vi "plcHMI.vi"() -> ()   [LabVIEW 2020]
doc: "ADS continuos synchronous write example using base blocks. \n\nThe client writes data synchronously and does wait for the respose from server."
uses:
  Agilent/AgilentTotalCluster.ctl
  Agilent/AgilentControl.ctl
  Agilent/Channel Config.ctl
  <vilib>/Platform/TimedLoop/XDataNode/timing_clust.ctl
  <vilib>/Platform/TimedLoop/XDataNode/nitl_modes.ctl
  <vilib>/Platform/TimedLoop/XDataNode/wakeup.ctl
  <userlib>/Beckhoff-LabVIEW-Interface/_DependsOn/With TypeResolving/Write Sync Single TypeResolved.vi
  <userlib>/Beckhoff-LabVIEW-Interface/_DependsOn/With TypeResolving/Read Sync Single TypeResolved.vi
  <vilib>/platform/TimedLoop/XDataNode/XDataNode.xnode
  <vilib>/Platform/TimedLoop/XDataNode/XDNodeRunTimeDep.lvlib
panel:
  in  "Tab Control":T1(tab)
  out "error out":errorcluster
  in  "Symbol file path - MUST BE ENTERED\nLoad \"ADS Write AND Read Symbols REV X.X.xml\"":path
  out "bHasMached":bool
  out "Write Status":bool
  out "Read Status":bool
  in  "EXIT HMI":bool caption="STOP HMI\nEXIT HMI"
  out "Internal TwinCAT Handle ID Maps":dbl format="%#_12g"
  in  "802L TDK PSU Voltage Rating (abs(Volts))":i32=12000 min=1 max=50000
  in  "802L TDL PSU Peak Power (J/s)":i32=9000 min=1 max=50000
  in  "HVPS Model":u16(ring) items=["802L-12kV,9000J/s", "802L+50kV,9000J/s", "Other"]
  in  "Voltage Held by PSU":bool
  in  "Log Capacitor Voltage":bool
  in  "Log Temperature Data":bool
  out "Time Since Last Shot":string caption="Elapsed Time Text"
  in  "Duty Cycle":dbl
  in  "Current Control":bool
  out "Expected Voltage":i16
  in  "Dump":bool
  out "EOC":bool
  out "Maximum Test Number Reached":bool
  out "SCR Ready":bool
  in  "START":bool
  in  "STOP":bool
  in  "Hold":bool
  in  "Charge":bool
  in  "Shot":bool
  in  "HV Switch Mode":bool
  in  "CLEAR FAULT":bool
  in  "Manual/Auto":bool=TRUE
  in  "Cycle Time (seconds)":i32=15 min=0
  in  "Capacitance (uF)":sgl=1e-13 min=0 max=10000 format="%#_6f"
  in  "Target Charge Volt (V) - Min 1500V - TEMPORARY LIMIT 12kV":i32 min=-12000 max=12000 step=1
  out "Estimated Charge Time (seconds)":sgl
  in  "Hold Time Before Shot (seconds)":i16 min=0 max=1000
  in  "Max Number of Shots (Test intervals)":i32=1 min=1 max=999
  out "Shot Number":i32
  out "Charge Fault":bool=TRUE
  out "Discharge Fault":bool=TRUE
  out "Hold Fault":bool=TRUE
  out "Cap 1 Temp\nExceeded Fault":bool=TRUE
  out "Ambient Temp\nExceeded Fault":bool=TRUE
  out "PSU Fault":bool=TRUE
  out "Control Sys Fault":bool=TRUE
  out "test Running":bool
  out "Test State":string
  out "Cap 1 Voltage":i16
  out "Cap 1 Temperature":i16
  in  "Capacitor Voltage Data Log File Path (.xlsx)":path
  out "Load Temperature":i16
  out "Soft Dump Temp":i16
  out "Ambient Temp":i16
  out "Waveform Chart - Capacitor Voltage (Probe, abs(Volts))":dbl(graph)
  in  "Manual Charge Time (seconds)":sgl=-1.0 min=-1 max=90
  in  "Reset Test Number":bool
  in  "Cap 1 Fault Temp (Cel)":i16 min=0 max=125
  in  "Capacitor Temperature Data Log File Path (.xlsx)":path
  out "Cap 1 Voltage (HVPS)":i16
  out "Capacitor Voltage":cluster{dbl, dbl}(graph)
  out "EOC":i16(graph)
  out "Soft Exception":bool
  out "PSU HV FB Fault":bool
  out "Charge FB Fault":bool
  out "Softdump FB Fault":bool
  out "SCR FB":i16(graph)
  in  "CH4 Vertical Units":string(combo)="V"
  in  "CH4 Vertical Units/div":dbl=2.0
  in  "Toggle Scope Scale":bool
  in  "CH1 Vertical Units/div":dbl=2.0
  in  "CH1 Vertical Units":string(combo)="V"
  in  "Horizontal Units":enum16{"us", "ms", "s"}(ring)
  in  "Horizontal Units/div":dbl=200.0
  out "Download":bool
  in  "Single":bool
  in  "Stop":bool
  out "Scope Trig":bool
  in  "Agilent Array":T2[](array[typedef])
  out "Process Step":i32
  out "Stop Loops":bool
  # "CONFIGURATION"
  # "Press STOP HMI instead of\nLabView Abort Execution"
  # "PSU V Rating, Peak Power\nactive when OTHER\nis selected"
  # "INPUT VARIABLES - For TDK Lambda 802L\nMust be written to before START"
  # "FAULT STATUSES"
  # "Set to -1 for automated\nfull charge to setpoint"
  # "MANUAL CONTROLS"
  # "Does not record during \"wait\" and appends to data file. Must be named with .xlsx"
  # "HV Switch Configuration"
  # "Records during \"Test Running.\" Must be named with .xlsx"
  # "Control Sys Faults"
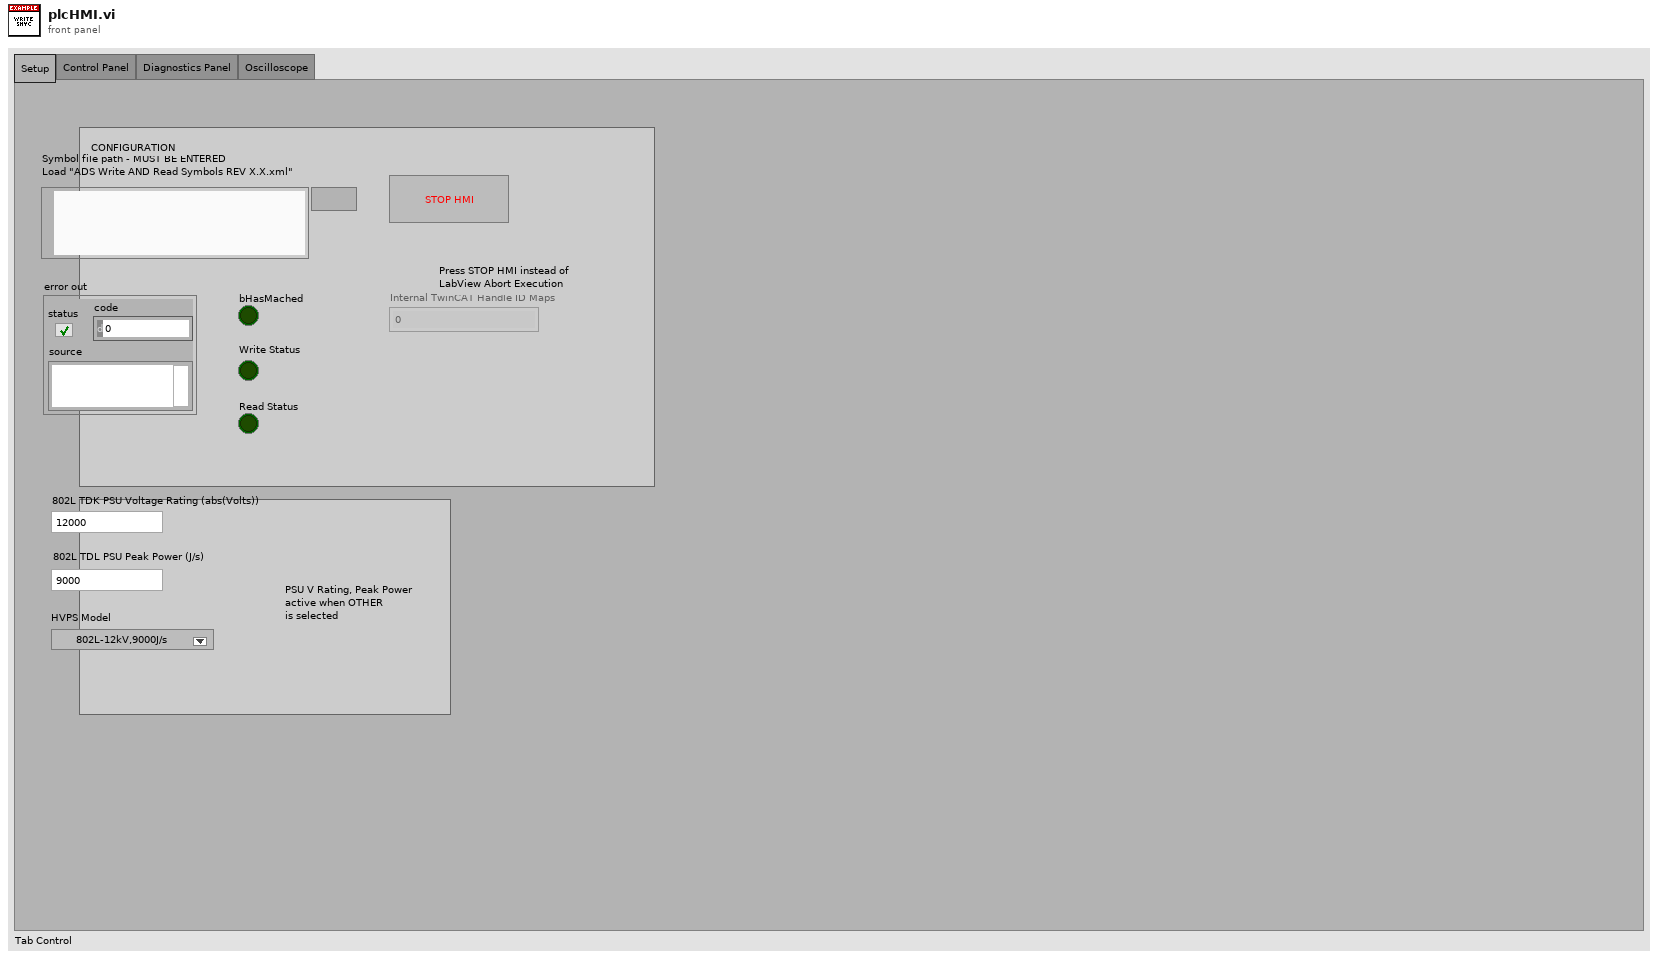
[diagram p1: front panel]
types:
  T1 = enum32{"Setup", "Control Panel", "Diagnostics Panel", "Oscilloscope"}
  T2 = typedef "AgilentTotalCluster.ctl" = cluster{"Agilent Graph":waveform(dbl)[], "Agilent Control":T3, "Agilent Setup Error":errorcluster, "Agilent Present":bool, "Enabled":bool}
  T3 = typedef "AgilentControl.ctl" = cluster{"Trig?":bool, "VISA session":refnum<visa-resource-name>, "Setup to Load":string, "Timeout (ms)":u32, "Desired Samp":enum32{"100", "250", "500", "1000", "2000", "5000", "10000", "20000", "50000", "100000", "200000", "500000", "1000000", "2000000", "4000000", "8000000"}, "Captured Samp":i32, "Desired Channels":T4[]}
  T4 = typedef "Channel Config.ctl" = cluster{"Chan Index":enum16{"Channel1", "Channel2", "Channel3", "Channel4", "MATH"}, "Name":string, "Samples":i32}
  T5 = typedef "XDNodeRunTimeDep.lvlib/timing_clust.ctl" = cluster{"Expected End [f-1]":u64, "Actual End [f-1]":u64, "Finished Late? [f-1]":bool, "Expected End [i-1]":u64, "Actual End [i-1]":u64, "Finished Late? [i-1]":bool, "Expected Start [i]":u64, "Actual Start [i]":u64, "Expected Start [f]":u64, "Actual Start [f]":u64, "Source Name":string, "Structure Name":string, "Period":i64, "Deadline":i64, "Offset":i64, "Start":i64, "Priority":i32, "Timeout":i32, "Mode":T6, "Wakeup Reason":T7, "Error":errorcluster, "Source Type":string, "Secondary Source Type":string, "Global End Time":u64, "Global Start Time":u64, "Frame Duration":u64, "Iteration Duration":u64, "Assigned CPU":i32, "I/O Scan Engine Mode":u32}
  T6 = typedef "XDNodeRunTimeDep.lvlib/nitl_modes.ctl" = enum32{"No Change", "Process missed periods, maintain original phase", "Discard missed periods, maintain original phase", "Process missed periods, ignore original phase", "Discard missed periods, ignore original phase"}
  T7 = typedef "XDNodeRunTimeDep.lvlib/wakeup.ctl" = enum32{"Normal", "Aborted", "Asynchronous wakeup", "Timing source error", "Timed loop error", "Timeout"}
  T8 = cluster{"Agilent Array[0]":T2, "Agilent Array[1]":T2, "Agilent Array[2]":T2, "Agilent Array[3]":T2, "Agilent Array[4]":T2, "Agilent Array[5]":T2, "Agilent Array[6]":T2, "Agilent Array[7]":T2, "Agilent Array[8]":T2}
  T9 = enum32{"100", "250", "500", "1000", "2000", "5000", "10000", "20000", "50000", "100000", "200000", "500000", "1000000", "2000000", "4000000", "8000000"}
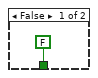
[diagram p2: hidden frame]
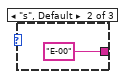
[diagram p5: hidden frame]
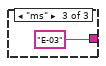
[diagram p6: hidden frame]
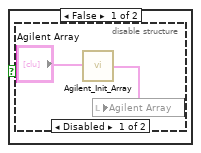
[diagram p7: hidden frame]
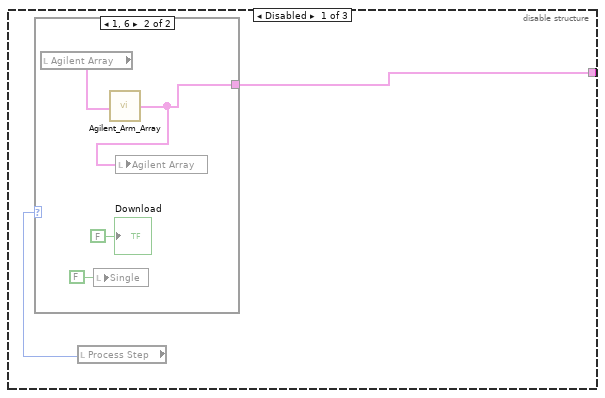
[diagram p11: hidden frame]
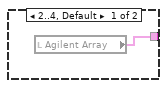
[diagram p12: hidden frame]
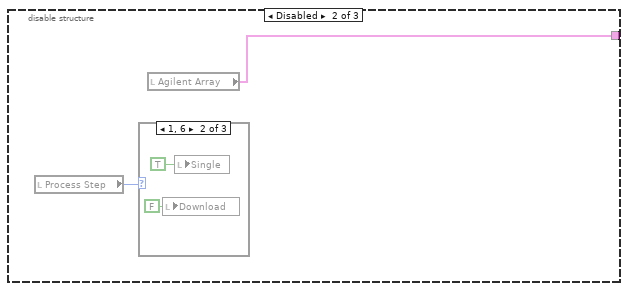
[diagram p13: hidden frame]
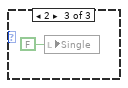
[diagram p15: hidden frame]
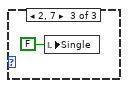
[diagram p17: hidden frame]
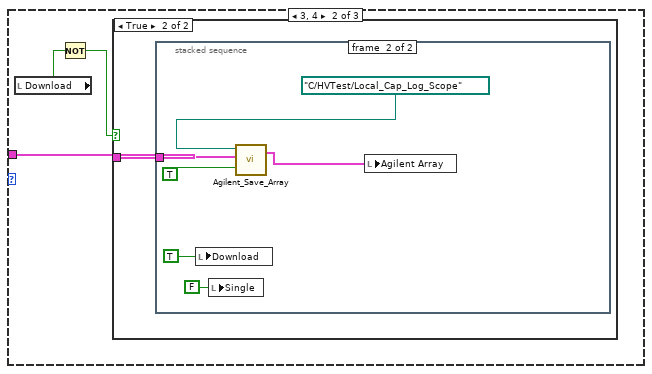
[diagram p19: hidden frame]
diagram:
  w89 = u16 17 items=["SyncLatest"=17, "AsyncLatest"=33] ("WriterMode")
  w182 = u16 33 items=["SyncLatest"=17, "AsyncLatest"=33] ("WriterMode")
  w221 = u16 33 items=["SyncLatest"=17, "AsyncLatest"=33] ("WriterMode")
  w240 = u16 33 items=["SyncLatest"=17, "AsyncLatest"=33] ("WriterMode")
  w259 = u16 33 items=["SyncLatest"=17, "AsyncLatest"=33] ("WriterMode")
  w278 = u16 33 items=["SyncLatest"=17, "AsyncLatest"=33] ("WriterMode")
  w297 = u16 33 items=["SyncLatest"=17, "AsyncLatest"=33] ("WriterMode")
  w316 = u16 33 items=["SyncLatest"=17, "AsyncLatest"=33] ("WriterMode")
  w335 = u16 17 items=["SyncLatest"=17, "AsyncLatest"=33] ("WriterMode")
  w354 = u16 17 items=["SyncLatest"=17, "AsyncLatest"=33] ("WriterMode")
  w373 = u16 17 items=["SyncLatest"=17, "AsyncLatest"=33] ("WriterMode")
  w392 = u16 17 items=["SyncLatest"=17, "AsyncLatest"=33] ("WriterMode")
  w411 = u16 17 items=["SyncLatest"=17, "AsyncLatest"=33] ("WriterMode")
  w430 = u16 17 items=["SyncLatest"=17, "AsyncLatest"=33] ("WriterMode")
  w449 = u16 17 items=["SyncLatest"=17, "AsyncLatest"=33] ("WriterMode")
  w464 = u16 17 items=["SyncLatest"=17, "AsyncLatest"=33] ("WriterMode")
  # "Variables/ Control"
  # "Documentation:\nCode separated vertically into two main sections - Write and read\nThey are further separated into BOOL and numeric\nThe OR gates wire all the error lines and the EXIT HMI button to a WHILE LOOP STOP\nThere current delay time on the routine is 100ms\nAll the AND gates connect the typecast resolve lines to the bHasMatched indicator\nThe second and third set of AND gates connect the write statuses to the Write Status indicator\nThe same is done for the read status indicator"
  # "WRITE NUMERICS"
  # "WRITE BOOLS"
  # "Select Symbol N"
  # "Read Initialization"
  # "Release \nTypeResolver"
  # "Release Writer"
  # "Send Request"
  # "Init \nTypeResolver"
  # "Init Writer"
  # "Select Symbol"
  # "Initialization"
  # "Call Release handle block\nat the end, when all nodes\nhave finished their execution"
  # "There must be only one release\nafter every init block.\nRelease block must be called\nalways at the end."
  # "Release"
  # "Symbol Interface"
  n1 = disable-structure shown="Enabled" {
    disable-tunnel: [w471 _] -> w469
    disable-tunnel: [w470 w473] -> w468
    frame Disabled {
      # "Using Symbol Interface"
      n2 = call <userlib>:"Symbol Interface.vi"() -> ("PortInfo"=w470:string, "error out"=w471:errorcluster)  [unwired: 14 in]
    }
    frame Enabled {
      # "Using Symbol File"
      n3 = Path To String(path="Symbol file path - MUST BE ENTERED\nLoad \"ADS Write AND Read Symbols REV X.X.xml\"") -> (string=w473:string)
    }
  }
  n4 = call <userlib>:"Init.vi"("XMLDescription"=w468, "error in (no error)"=w469) -> ("Handle"=w18:u32, "ReadGrpSymbols"=w16:string[], "WriteGrpSymbols"=w4:string[], "error out"=w9:errorcluster)  [unwired: 9 in, 1 out]
  n5 = Index Array(array=w4, index=21) -> (element=w3:string)
  n6 = Index Array(array=w4, index=20) -> (element=w10:string)
  n7 = Index Array(array=w4, index=14) -> (element=w222:string)
  n8 = Index Array(array=w4, index=9) -> (element=w317:string)
  n9 = Index Array(array=w4, index=10) -> (element=w298:string)
  n10 = Index Array(array=w4, index=12) -> (element=w260:string)
  n11 = Index Array(array=w4, index=11) -> (element=w279:string)
  n12 = Index Array(array=w4, index=13) -> (element=w241:string)
  n13 = Index Array(array=w4, index=18) -> (element=w19:string)
  n14 = Index Array(array=w4, index=19) -> (element=w11:string)
  n15 = Index Array(array=w4, index=7) -> (element=w336:string)
  n16 = Index Array(array=w4, index=2) -> (element=w431:string)
  n17 = Index Array(array=w4, index=3) -> (element=w412:string)
  n18 = Index Array(array=w4, index=5) -> (element=w374:string)
  n19 = Index Array(array=w4, index=4) -> (element=w393:string)
  n20 = Index Array(array=w4, index=6) -> (element=w355:string)
  n21 = Index Array(array=w4, index=1) -> (element=w450:string)
  n22 = Index Array(array=w4, index=16) -> (element=w116:string)
  n23 = Index Array(array=w4, index=8) -> (element=w88:string)
  n24 = Index Array(array=w4, index=0) -> (element=w465:string)
  n25 = Index Array(array=w4, index=15) -> (element=w183:string)
  n26 = Index Array(array=w4, index=17) -> (element=w72:string)
  n27 = call <userlib>:"Init Writer.vi"("Handle"=w18, "SymbolName"=w222, "WriterMode"=w221, "error constant"=w9) -> ("Handle"=w220:u32, "SymbolName"=w219:string, "WriterMode"=w218:u16, "WriteHandle"=w217:u32, "error IO"=w216:errorcluster)  [unwired: 7 in]
  n28 = call <userlib>:"Init Writer.vi"("Handle"=w18, "SymbolName"=w317, "WriterMode"=w316, "error constant"=w9) -> ("Handle"=w312:u32, "SymbolName"=w311:string, "WriterMode"=w310:u16, "WriteHandle"=w308:u32, "error IO"=w309:errorcluster)  [unwired: 7 in]
  n29 = call <userlib>:"Init Writer.vi"("Handle"=w18, "SymbolName"=w298, "WriterMode"=w297, "error constant"=w9) -> ("Handle"=w296:u32, "SymbolName"=w295:string, "WriterMode"=w294:u16, "WriteHandle"=w293:u32, "error IO"=w292:errorcluster)  [unwired: 7 in]
  n30 = call <userlib>:"Init Writer.vi"("Handle"=w18, "SymbolName"=w260, "WriterMode"=w259, "error constant"=w9) -> ("Handle"=w258:u32, "SymbolName"=w257:string, "WriterMode"=w256:u16, "WriteHandle"=w255:u32, "error IO"=w254:errorcluster)  [unwired: 7 in]
  n31 = call <userlib>:"Init Type.vi"("Handle"=w18, "SymbolName"=w222, "error in"=w9) -> ("Handle"=w215:u32, "TypeHdl"=w214:u32, "error IO"=w213:errorcluster)  [unwired: 7 in, 3 out]
  n32 = call <userlib>:"Init Type.vi"("Handle"=w18, "SymbolName"=w317, "error in"=w9) -> ("Handle"=w301:u32, "TypeHdl"=w300:u32, "error IO"=w299:errorcluster)  [unwired: 7 in, 3 out]
  n33 = call <userlib>:"Init Type.vi"("Handle"=w18, "SymbolName"=w298, "error in"=w9) -> ("Handle"=w291:u32, "TypeHdl"=w290:u32, "error IO"=w289:errorcluster)  [unwired: 7 in, 3 out]
  n34 = call <userlib>:"Init Writer.vi"("Handle"=w18, "SymbolName"=w279, "WriterMode"=w278, "error constant"=w9) -> ("Handle"=w277:u32, "SymbolName"=w276:string, "WriterMode"=w275:u16, "WriteHandle"=w274:u32, "error IO"=w273:errorcluster)  [unwired: 7 in]
  n35 = call <userlib>:"Init Type.vi"("Handle"=w18, "SymbolName"=w260, "error in"=w9) -> ("Handle"=w253:u32, "TypeHdl"=w252:u32, "error IO"=w251:errorcluster)  [unwired: 7 in, 3 out]
  n36 = call <userlib>:"Init Writer.vi"("Handle"=w18, "SymbolName"=w241, "WriterMode"=w240, "error constant"=w9) -> ("Handle"=w239:u32, "SymbolName"=w238:string, "WriterMode"=w237:u16, "WriteHandle"=w236:u32, "error IO"=w235:errorcluster)  [unwired: 7 in]
  n37 = call <userlib>:"Init Type.vi"("Handle"=w18, "SymbolName"=w279, "error in"=w9) -> ("Handle"=w272:u32, "TypeHdl"=w271:u32, "error IO"=w270:errorcluster)  [unwired: 7 in, 3 out]
  n38 = call <userlib>:"Init Type.vi"("Handle"=w18, "SymbolName"=w241, "error in"=w9) -> ("Handle"=w234:u32, "TypeHdl"=w233:u32, "error IO"=w232:errorcluster)  [unwired: 7 in, 3 out]
  n39 = call <userlib>:"Init Writer.vi"("Handle"=w18, "SymbolName"=w336, "WriterMode"=w335, "error constant"=w9) -> ("Handle"=w334:u32, "SymbolName"=w333:string, "WriterMode"=w332:u16, "WriteHandle"=w331:u32, "error IO"=w330:errorcluster)  [unwired: 7 in]
  n40 = call <userlib>:"Init Writer.vi"("Handle"=w18, "SymbolName"=w431, "WriterMode"=w430, "error constant"=w9) -> ("Handle"=w426:u32, "SymbolName"=w425:string, "WriterMode"=w424:u16, "WriteHandle"=w422:u32, "error IO"=w423:errorcluster)  [unwired: 7 in]
  n41 = call <userlib>:"Init Writer.vi"("Handle"=w18, "SymbolName"=w412, "WriterMode"=w411, "error constant"=w9) -> ("Handle"=w410:u32, "SymbolName"=w409:string, "WriterMode"=w408:u16, "WriteHandle"=w407:u32, "error IO"=w406:errorcluster)  [unwired: 7 in]
  n42 = call <userlib>:"Init Writer.vi"("Handle"=w18, "SymbolName"=w374, "WriterMode"=w373, "error constant"=w9) -> ("Handle"=w372:u32, "SymbolName"=w371:string, "WriterMode"=w370:u16, "WriteHandle"=w369:u32, "error IO"=w368:errorcluster)  [unwired: 7 in]
  n43 = call <userlib>:"Init Type.vi"("Handle"=w18, "SymbolName"=w336, "error in"=w9) -> ("Handle"=w329:u32, "TypeHdl"=w328:u32, "error IO"=w327:errorcluster)  [unwired: 7 in, 3 out]
  n44 = call <userlib>:"Init Type.vi"("Handle"=w18, "SymbolName"=w431, "error in"=w9) -> ("Handle"=w415:u32, "TypeHdl"=w414:u32, "error IO"=w413:errorcluster)  [unwired: 7 in, 3 out]
  n45 = call <userlib>:"Init Type.vi"("Handle"=w18, "SymbolName"=w412, "error in"=w9) -> ("Handle"=w405:u32, "TypeHdl"=w404:u32, "error IO"=w403:errorcluster)  [unwired: 7 in, 3 out]
  n46 = call <userlib>:"Init Writer.vi"("Handle"=w18, "SymbolName"=w393, "WriterMode"=w392, "error constant"=w9) -> ("Handle"=w391:u32, "SymbolName"=w390:string, "WriterMode"=w389:u16, "WriteHandle"=w388:u32, "error IO"=w387:errorcluster)  [unwired: 7 in]
  n47 = call <userlib>:"Init Type.vi"("Handle"=w18, "SymbolName"=w374, "error in"=w9) -> ("Handle"=w367:u32, "TypeHdl"=w366:u32, "error IO"=w365:errorcluster)  [unwired: 7 in, 3 out]
  n48 = call <userlib>:"Init Writer.vi"("Handle"=w18, "SymbolName"=w355, "WriterMode"=w354, "error constant"=w9) -> ("Handle"=w353:u32, "SymbolName"=w352:string, "WriterMode"=w351:u16, "WriteHandle"=w350:u32, "error IO"=w349:errorcluster)  [unwired: 7 in]
  n49 = call <userlib>:"Init Type.vi"("Handle"=w18, "SymbolName"=w393, "error in"=w9) -> ("Handle"=w386:u32, "TypeHdl"=w385:u32, "error IO"=w384:errorcluster)  [unwired: 7 in, 3 out]
  n50 = call <userlib>:"Init Type.vi"("Handle"=w18, "SymbolName"=w355, "error in"=w9) -> ("Handle"=w348:u32, "TypeHdl"=w347:u32, "error IO"=w346:errorcluster)  [unwired: 7 in, 3 out]
  n51 = call <userlib>:"Init Writer.vi"("Handle"=w18, "SymbolName"=w450, "WriterMode"=w449, "error constant"=w9) -> ("Handle"=w448:u32, "SymbolName"=w447:string, "WriterMode"=w446:u16, "WriteHandle"=w445:u32, "error IO"=w444:errorcluster)  [unwired: 7 in]
  n52 = call <userlib>:"Init Writer.vi"("Handle"=w18, "SymbolName"=w116, "error constant"=w9) -> ("Handle"=w115:u32, "SymbolName"=w114:string, "WriterMode"=w113:u16, "WriteHandle"=w111:u32, "error IO"=w112:errorcluster)  [unwired: 8 in]
  n53 = call <userlib>:"Init Type.vi"("Handle"=w18, "SymbolName"=w450, "error in"=w9) -> ("Handle"=w443:u32, "TypeHdl"=w442:u32, "error IO"=w441:errorcluster)  [unwired: 7 in, 3 out]
  n54 = call <userlib>:"Init Type.vi"("Handle"=w18, "SymbolName"=w116, "error in"=w9) -> ("Handle"=w110:u32, "TypeHdl"=w109:u32, "error IO"=w108:errorcluster)  [unwired: 7 in, 3 out]
  n55 = call <userlib>:"Init Writer.vi"("Handle"=w18, "SymbolName"=w465, "WriterMode"=w464, "error constant"=w9) -> ("Handle"=w463:u32, "SymbolName"=w462:string, "WriterMode"=w461:u16, "WriteHandle"=w460:u32, "error IO"=w459:errorcluster)  [unwired: 7 in]
  n56 = call <userlib>:"Init Type.vi"("Handle"=w18, "SymbolName"=w465, "error in"=w9) -> ("Handle"=w458:u32, "TypeHdl"=w457:u32, "error IO"=w452:errorcluster)  [unwired: 7 in, 3 out]
  n57 = call <userlib>:"Init Writer.vi"("Handle"=w18, "SymbolName"=w183, "WriterMode"=w182, "error constant"=w9) -> ("Handle"=w178:u32, "SymbolName"=w177:string, "WriterMode"=w176:u16, "WriteHandle"=w165:u32, "error IO"=w175:errorcluster)  [unwired: 7 in]
  n58 = call <userlib>:"Init Type.vi"("Handle"=w18, "SymbolName"=w183, "error in"=w9) -> ("Handle"=w171:u32, "TypeHdl"=w169:u32, "error IO"=w170:errorcluster)  [unwired: 7 in, 3 out]
  n59 = call <userlib>:"Init Writer.vi"("Handle"=w18, "SymbolName"=w72, "error constant"=w9) -> ("Handle"=w69:u32, "SymbolName"=w68:string, "WriterMode"=w67:u16, "WriteHandle"=w66:u32, "error IO"=w65:errorcluster)  [unwired: 8 in]
  n60 = call <userlib>:"Init Type.vi"("Handle"=w18, "SymbolName"=w72, "error in"=w9) -> ("Handle"=w64:u32, "TypeHdl"=w63:u32, "error IO"=w62:errorcluster)  [unwired: 7 in, 3 out]
  n61 = Index Array(array=w16, index=2) -> (element=w161:string)
  n62 = Index Array(array=w16, index=4) -> (element=w157:string)
  n63 = call <userlib>:"Init Writer.vi"("Handle"=w18, "SymbolName"=w88, "WriterMode"=w89, "error constant"=w9) -> ("Handle"=w87:u32, "SymbolName"=w86:string, "WriterMode"=w85:u16, "WriteHandle"=w84:u32, "error IO"=w83:errorcluster)  [unwired: 7 in]
  n64 = Index Array(array=w16, index=1) -> (element=w200:string)
  n65 = Index Array(array=w16, index=21) -> (element=w33:string)
  n66 = Index Array(array=w16, index=22) -> (element=w30:string)
  n67 = call <userlib>:"Init Type.vi"("Handle"=w18, "SymbolName"=w88, "error in"=w9) -> ("Handle"=w82:u32, "TypeHdl"=w81:u32, "error IO"=w80:errorcluster)  [unwired: 7 in, 3 out]
  n68 = Index Array(array=w16, index=0) -> (element=w199:string)
  n69 = Index Array(array=w16, index=3) -> (element=w158:string)
  n70 = Index Array(array=w16, index=20) -> (element=w38:string)
  n71 = Index Array(array=w16, index=23) -> (element=w29:string)
  n72 = Index Array(array=w16, index=16) -> (element=w163:string)
  n73 = Index Array(array=w16, index=24) -> (element=w27:string)
  n74 = Index Array(array=w16, index=11) -> (element=w188:string)
  n75 = Index Array(array=w16, index=10) -> (element=w189:string)
  n76 = Index Array(array=w16, index=17) -> (element=w41:string)
  n77 = Index Array(array=w16, index=18) -> (element=w40:string)
  n78 = Index Array(array=w16, index=13) -> (element=w186:string)
  n79 = Index Array(array=w16, index=12) -> (element=w187:string)
  n80 = Index Array(array=w16, index=15) -> (element=w184:string)
  n81 = Index Array(array=w16, index=19) -> (element=w39:string)
  n82 = Index Array(array=w16, index=5) -> (element=w53:string)
  n83 = Index Array(array=w16, index=6) -> (element=w151:string)
  n84 = Index Array(array=w16, index=9) -> (element=w198:string)
  n85 = Index Array(array=w16, index=14) -> (element=w185:string)
  n86 = Index Array(array=w16, index=8) -> (element=w153:string)
  n87 = Index Array(array=w16, index=25) -> (element=w15:string)
  n88 = Index Array(array=w16, index=7) -> (element=w152:string)
  n89 = node-c288(10) -> (w98:T5)  [unwired: 3 in]
  n90 = timed-loop {
    tunnel: w463 -> [w771]
    tunnel: w462 -> [w770]
    tunnel: w461 -> [w769]
    tunnel: w460 -> [w768]
    tunnel: w458 -> [w1045]
    tunnel: w457 -> [w1044]
    tunnel: [w766] -> w456
    tunnel: [w765] -> w455
    tunnel: [w1043] -> w454
    tunnel: [w1042] -> w453
    tunnel: w448 -> [w1040]
    tunnel: w447 -> [w1039]
    tunnel: w446 -> [w1038]
    tunnel: w445 -> [w1037]
    tunnel: w443 -> [w1035]
    tunnel: w442 -> [w1034]
    tunnel: [w1032] -> w439
    tunnel: [w1031] -> w438
    tunnel: [w1030] -> w436
    tunnel: [w1029] -> w435
    tunnel: w426 -> [w1028]
    tunnel: w425 -> [w1027]
    tunnel: w424 -> [w1026]
    tunnel: w422 -> [w1024]
    tunnel: [w1023] -> w421
    tunnel: [w1022] -> w420
    tunnel: [w1021] -> w417
    tunnel: [w1020] -> w416
    tunnel: w415 -> [w1019]
    tunnel: w414 -> [w1018]
    tunnel: w410 -> [w1016]
    tunnel: w409 -> [w1015]
    tunnel: w408 -> [w1014]
    tunnel: w407 -> [w1013]
    tunnel: w405 -> [w1011]
    tunnel: w404 -> [w1010]
    tunnel: [w1008] -> w401
    tunnel: [w1007] -> w400
    tunnel: [w1006] -> w398
    tunnel: [w1005] -> w397
    tunnel: w391 -> [w1004]
    tunnel: w390 -> [w1003]
    tunnel: w389 -> [w1002]
    tunnel: w388 -> [w1001]
    tunnel: w386 -> [w999]
    tunnel: w385 -> [w998]
    tunnel: [w996] -> w382
    tunnel: [w995] -> w381
    tunnel: [w994] -> w379
    tunnel: [w993] -> w378
    tunnel: w372 -> [w992]
    tunnel: w371 -> [w991]
    tunnel: w370 -> [w990]
    tunnel: w369 -> [w989]
    tunnel: w367 -> [w987]
    tunnel: w366 -> [w986]
    tunnel: [w984] -> w363
    tunnel: [w983] -> w362
    tunnel: [w982] -> w360
    tunnel: [w981] -> w359
    tunnel: w353 -> [w980]
    tunnel: w352 -> [w979]
    tunnel: w351 -> [w978]
    tunnel: w350 -> [w977]
    tunnel: w348 -> [w975]
    tunnel: w347 -> [w974]
    tunnel: [w972] -> w344
    tunnel: [w971] -> w343
    tunnel: [w970] -> w341
    tunnel: [w969] -> w340
    tunnel: w334 -> [w968]
    tunnel: w333 -> [w967]
    tunnel: w332 -> [w966]
    tunnel: w331 -> [w965]
    tunnel: w329 -> [w963]
    tunnel: w328 -> [w962]
    tunnel: [w960] -> w325
    tunnel: [w959] -> w324
    tunnel: [w958] -> w322
    tunnel: [w957] -> w321
    tunnel: w312 -> [w956]
    tunnel: w311 -> [w955]
    tunnel: w310 -> [w954]
    tunnel: w308 -> [w952]
    tunnel: [w951] -> w307
    tunnel: [w950] -> w306
    tunnel: [w949] -> w303
    tunnel: [w948] -> w302
    tunnel: w301 -> [w947]
    tunnel: w300 -> [w946]
    tunnel: w296 -> [w944]
    tunnel: w295 -> [w943]
    tunnel: w294 -> [w942]
    tunnel: w293 -> [w941]
    tunnel: w291 -> [w939]
    tunnel: w290 -> [w938]
    tunnel: [w936] -> w287
    tunnel: [w935] -> w286
    tunnel: [w934] -> w284
    tunnel: [w933] -> w283
    tunnel: w277 -> [w932]
    tunnel: w276 -> [w931]
    tunnel: w275 -> [w930]
    tunnel: w274 -> [w929]
    tunnel: w272 -> [w927]
    tunnel: w271 -> [w926]
    tunnel: [w924] -> w268
    tunnel: [w923] -> w267
    tunnel: [w922] -> w265
    tunnel: [w921] -> w264
    tunnel: w258 -> [w920]
    tunnel: w257 -> [w919]
    tunnel: w256 -> [w918]
    tunnel: w255 -> [w917]
    tunnel: w253 -> [w915]
    tunnel: w252 -> [w914]
    tunnel: [w912] -> w249
    tunnel: [w911] -> w248
    tunnel: [w910] -> w246
    tunnel: [w909] -> w245
    tunnel: w239 -> [w908]
    tunnel: w238 -> [w907]
    tunnel: w237 -> [w906]
    tunnel: w236 -> [w905]
    tunnel: w234 -> [w903]
    tunnel: w233 -> [w902]
    tunnel: [w900] -> w230
    tunnel: [w899] -> w229
    tunnel: [w898] -> w227
    tunnel: [w897] -> w226
    tunnel: w220 -> [w896]
    tunnel: w219 -> [w895]
    tunnel: w218 -> [w894]
    tunnel: w217 -> [w893]
    tunnel: w215 -> [w891]
    tunnel: w214 -> [w890]
    tunnel: [w888] -> w211
    tunnel: [w887] -> w210
    tunnel: [w886] -> w208
    tunnel: [w885] -> w207
    tunnel: w200 -> [w884]
    tunnel: w199 -> [w883]
    tunnel: w198 -> [w882]
    tunnel: [w881] -> w146
    tunnel: w189 -> [w880]
    tunnel: w188 -> [w879]
    tunnel: w187 -> [w878]
    tunnel: w186 -> [w877]
    tunnel: w185 -> [w876]
    tunnel: w184 -> [w875]
    tunnel: [w874] -> w94
    tunnel: [w873] -> w145
    tunnel: [w872] -> w144
    tunnel: [w871] -> w143
    tunnel: [w870] -> w142
    tunnel: [w812] -> w141
    tunnel: [w810] -> w140
    shift-right: [w694] -> w467
    shift-left: w459 -> [w767]
    shift-right: [w693] -> w466
    shift-left: w452 -> [w1041]
    shift-right: [w691] -> w437
    shift-left: w444 -> [w1036]
    shift-right: [w690] -> w434
    shift-left: w441 -> [w1033]
    shift-right: [w688] -> w419
    shift-left: w423 -> [w1025]
    shift-right: [w687] -> w418
    shift-left: w413 -> [w1017]
    shift-right: [w685] -> w399
    shift-left: w406 -> [w1012]
    shift-right: [w684] -> w396
    shift-left: w403 -> [w1009]
    shift-right: [w682] -> w380
    shift-left: w387 -> [w1000]
    shift-right: [w681] -> w377
    shift-left: w384 -> [w997]
    shift-right: [w679] -> w361
    shift-left: w368 -> [w988]
    shift-right: [w678] -> w358
    shift-left: w365 -> [w985]
    shift-right: [w676] -> w342
    shift-left: w349 -> [w976]
    shift-right: [w675] -> w339
    shift-left: w346 -> [w973]
    shift-right: [w673] -> w323
    shift-left: w330 -> [w964]
    shift-right: [w672] -> w320
    shift-left: w327 -> [w961]
    shift-right: [w671] -> w305
    shift-left: w309 -> [w953]
    shift-right: [w670] -> w304
    shift-left: w299 -> [w945]
    shift-right: [w668] -> w285
    shift-left: w292 -> [w940]
    shift-right: [w667] -> w282
    shift-left: w289 -> [w937]
    shift-right: [w665] -> w266
    shift-left: w273 -> [w928]
    shift-right: [w664] -> w263
    shift-left: w270 -> [w925]
    shift-right: [w662] -> w247
    shift-left: w254 -> [w916]
    shift-right: [w661] -> w244
    shift-left: w251 -> [w913]
    shift-right: [w659] -> w228
    shift-left: w235 -> [w904]
    shift-right: [w658] -> w225
    shift-left: w232 -> [w901]
    shift-right: [w656] -> w209
    shift-left: w216 -> [w892]
    shift-right: [w655] -> w206
    shift-left: w213 -> [w889]
    tunnel: w178 -> [w852]
    tunnel: w177 -> [w851]
    tunnel: w176 -> [w850]
    tunnel: w175 -> [w849]
    tunnel: [w653] -> w174
    tunnel: [w848] -> w173
    tunnel: [w847] -> w172
    tunnel: w171 -> [w846]
    tunnel: w170 -> [w845]
    tunnel: w169 -> [w844]
    tunnel: [w652] -> w168
    tunnel: [w843] -> w167
    tunnel: [w842] -> w166
    tunnel: w165 -> [w841]
    tunnel: w163 -> [w840]
    tunnel: [w811] -> w139
    tunnel: [w834] -> w148
    tunnel: w9 -> [w833]
    tunnel: [w831] -> w147
    tunnel: w161 -> [w830]
    tunnel: w158 -> [w826]
    tunnel: w157 -> [w825]
    tunnel: [w816] -> w149
    tunnel: [w815] -> w150
    tunnel: w153 -> [w809]
    tunnel: w152 -> [w808]
    tunnel: w151 -> [w807]
    tunnel: [w794] -> w50
    tunnel: [w793] -> w49
    tunnel: [w792] -> w48
    tunnel: w115 -> [w785]
    tunnel: w114 -> [w784]
    tunnel: w113 -> [w783]
    tunnel: w112 -> [w782]
    tunnel: w111 -> [w781]
    tunnel: w110 -> [w779]
    tunnel: w109 -> [w778]
    tunnel: w108 -> [w777]
    tunnel: [w776] -> w105
    tunnel: [w775] -> w104
    tunnel: [w650] -> w103
    tunnel: [w649] -> w102
    tunnel: [w774] -> w101
    tunnel: [w773] -> w100
    timing: w98 -> [_]
    timing-out: [_] -> w97
    tunnel: w18 -> [w764]
    tunnel: [w647] -> w52
    tunnel: w87 -> [w642]
    tunnel: w86 -> [w641]
    tunnel: w85 -> [w640]
    tunnel: w84 -> [w639]
    tunnel: w83 -> [w638]
    tunnel: w82 -> [w637]
    tunnel: w81 -> [w636]
    tunnel: w80 -> [w635]
    tunnel: [w633] -> w79
    tunnel: [w632] -> w78
    tunnel: [w625] -> w77
    tunnel: [w624] -> w76
    tunnel: [w631] -> w75
    tunnel: [w630] -> w74
    tunnel: w69 -> [w618]
    tunnel: w68 -> [w617]
    tunnel: w67 -> [w616]
    tunnel: w66 -> [w615]
    tunnel: w65 -> [w614]
    tunnel: w64 -> [w613]
    tunnel: w63 -> [w612]
    tunnel: w62 -> [w611]
    tunnel: [w609] -> w61
    tunnel: [w606] -> w60
    tunnel: [w601] -> w59
    tunnel: [w600] -> w58
    tunnel: [w608] -> w57
    tunnel: [w607] -> w56
    tunnel: [w599] -> w51
    tunnel: w53 -> [w595]
    tunnel: [w594] -> w47
    tunnel: w41 -> [w588]
    tunnel: w40 -> [w583]
    tunnel: w39 -> [w582]
    tunnel: w38 -> [w581]
    tunnel: [w578] -> w37
    tunnel: [w576] -> w36
    tunnel: [w571] -> w35
    tunnel: [w570] -> w22
    tunnel: w33 -> [w568]
    tunnel: w30 -> [w543]
    tunnel: w29 -> [w542]
    tunnel: w27 -> [w535]
    tunnel: [w531] -> w26
    tunnel: [w530] -> w25
    tunnel: [w529] -> w24
    tunnel: [w528] -> w23
    tunnel: w19 -> [w527]
    tunnel: w18 -> [w489]
    tunnel: w9 -> [w526]
    tunnel: [w521] -> w8
    tunnel: [w520] -> _
    tunnel: w15 -> [w516]
    tunnel: [w512] -> w14
    tunnel: w11 -> [w511]
    tunnel: w10 -> [w510]
    tunnel: w9 -> [w485]
    tunnel: [w505] -> w7
    tunnel: [w504] -> w6
    tunnel: w3 -> [w490]
    tunnel: [w484] -> w2
    stop <- w589 stop-if-true
    # "Stop Loop on Error (OR gates)"
    # "Error Stop Loop AND"
    # "Typecast Match AND"
    # "Write Status AND"
    # "READ BOOLS"
    # "READ NUMERICS"
    # "STOP HMI via error or EXIT button"
    # "Check Read status and\nthen convert Variant \nto LabVIEW type (AND gates)"
    # "Sync Read Single"
    n91 = node-c288() -> (w648:errorcluster)  [unwired: 1 in]
    n92 = disable-structure shown="Enabled" {
      frame Enabled {
        n93 = flat-sequence {
          tunnel: [w1185] -> w1129
          tunnel: w1129 -> [w1204]
          frame #0 {
            n94 = disable-structure shown="Enabled" {
              frame Enabled {
                n95 = feedback #1(TRUE) -> (w1131:bool)
                n96 = And(x=TRUE, y=w1131) -> (x .and. y?=w1134:bool)
                n97 = case shown="True" w1134 {
                  tunnel: [FALSE FALSE] -> w1132
                  frame False {
                  }
                  frame True {
                    n98 = local read "Agilent Array"() -> (w1137:T2[])
                    n99 = call "Agilent_Init_Array.vi"("Agilent Array In"=w1137) -> ("Agilent Array Out"=w1138:T2[])
                    n100 = call "Agilent_Arm_Array.vi"("Agilent Array In"=w1138) -> ("Agilent Array Out"=w1136:T2[])
                    n101 = local write "Agilent Array"(w1136) -> ()
                  }
                }
                n102 = feedback-in #1(w1132) -> ()
              }
              frame Disabled {
              }
            }
          }
          frame #1 {
            n103 = case shown="True" "Toggle Scope Scale" {
              frame False {
              }
              frame True {
                n104 = Number To Decimal String(number="CH4 Vertical Units/div") -> (decimal integer string=w1144:string)  [unwired: 1 in]
                n105 = Number To Decimal String(number="Horizontal Units/div") -> (decimal integer string=w1152:string)  [unwired: 1 in]
                n106 = Number To Decimal String(number="CH1 Vertical Units/div") -> (decimal integer string=w1150:string)  [unwired: 1 in]
                n107 = case shown="\"us\"" "Horizontal Units" {
                  tunnel: ["E-06" "E-00" "E-03"] -> w1161
                  frame "us" {
                  }
                  frame "s", Default {
                  }
                  frame "ms" {
                  }
                }
                n108 = Concatenate Strings(":CHAN4:SCAL " ("write buffer"), w1144, "CH4 Vertical Units") -> (w1143:string)
                n109 = Concatenate Strings(":CHAN1:SCAL " ("write buffer"), w1150, "CH1 Vertical Units") -> (w1157:string)
                n110 = Concatenate Strings(":TIM:SCAL " ("write buffer"), w1152, w1161) -> (w1160:string)
                n111 = VISA Open(VISA resource name=refnum<visa-resource-name> "HV_Test_Scope") -> (VISA resource name=w1155:refnum<visa-resource-name>, error out=w1156:errorcluster)  [unwired: 4 in]
                n112 = VISA Write(VISA resource name=w1155, write buffer=w1160, error in (no error)=w1156) -> (VISA resource name out=w1164:refnum<visa-resource-name>, error out=w1163:errorcluster)  [unwired: 1 out]
                n113 = VISA Write(VISA resource name=w1164, write buffer=w1157, error in (no error)=w1163) -> (VISA resource name out=w1149:refnum<visa-resource-name>, error out=w1147:errorcluster)  [unwired: 1 out]
                n114 = VISA Write(VISA resource name=w1149, write buffer=w1143, error in (no error)=w1147) -> (VISA resource name out=w1148:refnum<visa-resource-name>, error out=w1146:errorcluster)  [unwired: 1 out]
                n115 = VISA Close(VISA resource name=w1148, error in (no error)=w1146) -> ()  [unwired: 1 out]
              }
            }
          }
          frame #2 {
            n116 = disable-structure shown="Enabled" {
              frame Enabled {
                n117 = case shown="True" "Stop" {
                  frame False {
                    n118 = disable-structure shown="Disabled" {
                      frame Disabled {
                        n119 = call "Agilent_Init_Array.vi"("Agilent Array In"="Agilent Array") -> ("Agilent Array Out"=w1171:T2[])
                        n120 = local write "Agilent Array"(w1171) -> ()
                      }
                      frame Enabled {
                      }
                    }
                  }
                  frame True {
                    n121 = VISA Open(VISA resource name=refnum<visa-resource-name> "HV_Test_Scope") -> (VISA resource name=w1177:refnum<visa-resource-name>, error out=w1178:errorcluster)  [unwired: 4 in]
                    n122 = VISA Write(VISA resource name=w1177, write buffer=":STOP", error in (no error)=w1178) -> (VISA resource name out=w1175:refnum<visa-resource-name>, error out=w1176:errorcluster)  [unwired: 1 out]
                    n123 = VISA Close(VISA resource name=w1175, error in (no error)=w1176) -> ()  [unwired: 1 out]
                  }
                }
              }
              frame Disabled {
              }
            }
            n124 = case shown="True" "Single" {
              frame False {
              }
              frame True {
                n125 = VISA Open(VISA resource name=refnum<visa-resource-name> "HV_Test_Scope") -> (VISA resource name=w1183:refnum<visa-resource-name>, error out=w1184:errorcluster)  [unwired: 4 in]
                n126 = VISA Write(VISA resource name=w1183, write buffer=":SINGLE", error in (no error)=w1184) -> (VISA resource name out=w1181:refnum<visa-resource-name>, error out=w1182:errorcluster)  [unwired: 1 out]
                n127 = VISA Close(VISA resource name=w1181, error in (no error)=w1182) -> ()  [unwired: 1 out]
              }
            }
          }
          frame #3 {
            n128 = disable-structure shown="Enabled" {
              disable-tunnel: [w1187 w1194 w1199] -> w1185
              frame Disabled {
                n129 = local read "Process Step"() -> (w1186:i32)
                n130 = case shown="1, 6" w1186 {
                  tunnel: [w1188 w1192] -> w1187
                  frame 2..4, Default {
                    n131 = local read "Agilent Array"() -> (w1188:T2[])
                  }
                  frame 1, 6 {
                    n132 = local read "Agilent Array"() -> (w1189:T2[])
                    n133 = local write "Single"(FALSE ("Single")) -> ()
                    n134 = call "Agilent_Arm_Array.vi"("Agilent Array In"=w1189) -> ("Agilent Array Out"=w1192:T2[])
                    n135 = local write "Agilent Array"(w1192) -> ()
                    "Download" <- FALSE ("Downloading")
                  }
                }
              }
              frame Disabled {
                n136 = local read "Process Step"() -> (w1193:i32)
                n137 = case shown="1, 6" w1193 {
                  frame 0, Default {
                  }
                  frame 1, 6 {
                    n138 = local write "Download"(FALSE ("Download")) -> ()
                    n139 = local write "Single"(TRUE ("Single")) -> ()
                  }
                  frame 2 {
                    n140 = local write "Single"(FALSE ("Single")) -> ()
                  }
                }
                n141 = local read "Agilent Array"() -> (w1194:T2[])
              }
              frame Enabled {
                n142 = local read "Process Step"() -> (w1198:i32)
                n143 = case shown="1, 6" w1198 {
                  frame 0, Default {
                  }
                  frame 1, 6 {
                    n144 = local write "Download"(FALSE ("Download")) -> ()
                    n145 = local write "Single"(TRUE ("Single")) -> ()
                  }
                  frame 2, 7 {
                    n146 = local write "Single"(FALSE ("Single")) -> ()
                  }
                }
                n147 = local read "Agilent Array"() -> (w1199:T2[])
              }
            }
          }
          frame #4 {
            n148 = local read "Process Step"() -> (w1203:i32)
            n149 = case shown="0" w1203 {
              tunnel: w1204 -> [_ w1207 w1220]
              frame Default {
              }
              frame 3, 4 {
                n150 = local read "Download"() -> (w1206:bool)
                n151 = Not(x=w1206) -> (.not. x?=w1205:bool)
                n152 = case shown="True" w1205 {
                  tunnel: w1207 -> [_ w1208]
                  frame False {
                  }
                  frame True {
                    n153 = stacked-sequence {
                      tunnel: w1208 -> [_ w1218]
                      frame #0 {
                        n154 = local read "Agilent Array"() -> (w1212:T2[])
                        n155 = Array To Cluster(array=w1212) -> (cluster=w1211:T8)
                        n156 = Unbundle By Name(w1211) -> ("Agilent Array[0].Agilent Control.Desired Samp"=w1209:T9)
                        n157 = call "GF_SetRecordLengthProperly.vi"("Num Samples"=w1209, "VISA resource name"=refnum<visa-resource-name> "HV_Test_Scope") -> ()  [unwired: 1 in, 2 out]
                      }
                      frame #1 {
                        n158 = local write "Download"(TRUE ("Downloading")) -> ()
                        n159 = local write "Single"(FALSE ("Single")) -> ()
                        n160 = call "Agilent_Save_Array.vi"("Agilent Download"=TRUE, "Agilent Array In"=w1218, "File Path"=path "C:/HVTest/Local_Cap_Log_Scope") -> ("Agilent Array Out"=w1216:T2[])  [unwired: 1 in, 1 out]
                        n161 = local write "Agilent Array"(w1216) -> ()
                      }
                    }
                  }
                }
              }
              frame 0 {
                n162 = local read "Maximum Test Number Reached"() -> (w1219:bool)
                n163 = case shown="True" w1219 {
                  tunnel: w1220 -> [_ w1223]
                  frame False {
                  }
                  frame True {
                    n164 = local read "Download"() -> (w1222:bool)
                    n165 = Not(x=w1222) -> (.not. x?=w1221:bool)
                    n166 = case shown="True" w1221 {
                      tunnel: w1223 -> [_ w1224]
                      frame False {
                      }
                      frame True {
                        n167 = stacked-sequence {
                          tunnel: w1224 -> [_ w1234]
                          frame #0 {
                            n168 = local read "Agilent Array"() -> (w1228:T2[])
                            n169 = Array To Cluster(array=w1228) -> (cluster=w1227:T8)
                            n170 = Unbundle By Name(w1227) -> ("Agilent Array[0].Agilent Control.Desired Samp"=w1225:T9)
                            n171 = call "GF_SetRecordLengthProperly.vi"("Num Samples"=w1225, "VISA resource name"=refnum<visa-resource-name> "HV_Test_Scope") -> ()  [unwired: 1 in, 2 out]
                          }
                          frame #1 {
                            n172 = local write "Download"(TRUE ("Downloading")) -> ()
                            n173 = local write "Single"(FALSE ("Single")) -> ()
                            n174 = call "Agilent_Save_Array.vi"("Agilent Download"=TRUE, "Agilent Array In"=w1234, "File Path"=path "C:/HVTest/Local_Cap_Log_Scope") -> ("Agilent Array Out"=w1232:T2[])  [unwired: 1 in, 1 out]
                            n175 = local write "Agilent Array"(w1232) -> ()
                          }
                        }
                      }
                    }
                  }
                }
              }
            }
          }
        }
      }
      frame Disabled {
      }
    }
    n176 = case shown="0, Default" "HVPS Model" {
      tunnel: ["802L TDK PSU Voltage Rating (abs(Volts))" 12000 50000] -> w772
      tunnel: ["802L TDL PSU Peak Power (J/s)" 9000 9000] -> w813
      frame 2 {
      }
      frame 0, Default {
      }
      frame 1 {
      }
    }
    n177 = flat-sequence {
      tunnel: w613 -> [w1255]
      tunnel: w612 -> [w1256]
      tunnel: w611 -> [w1253]
      tunnel: [w1253] -> w622
      tunnel: [w1256] -> w621
      tunnel: [w1255] -> w620
      tunnel: [w1254] -> w619
      tunnel: [w1259] -> w600
      tunnel: [w1262] -> w607
      tunnel: [w1261] -> w608
      tunnel: [w1260] -> w610
      tunnel: w622 -> [w1265]
      tunnel: w621 -> [w1264]
      tunnel: w620 -> [w1263]
      tunnel: w619 -> [w1258]
      tunnel: [w1257] -> w523
      frame #0 {
        # "Write Data"
        n178 = To Word Integer(number="Cap 1 Fault Temp (Cel)") -> (16bit integer=w1251:i16)
        n179 = To Variant(anything=w1251) -> (Variant=w1254:variant)
      }
      frame #1 {
        # "Resolve To TC"
        n180 = call <userlib>:"Resolve To TC Type.vi"("Handle"=w1263, "TypHdl"=w1264, "WData"=w1258, "error in"=w1265) -> ("Handle"=w1261:u32, "TypHdl"=w1262:u32, "bHasMatched"=w1257:bool, "ADSWData"=w1260:variant, "error out"=w1259:errorcluster)  [unwired: 7 in]
      }
    }
    n181 = flat-sequence {
      tunnel: w891 -> [w1467]
      tunnel: w890 -> [w1468]
      tunnel: w889 -> [w1469]
      tunnel: [w1469] -> w1073
      tunnel: [w1468] -> w1072
      tunnel: [w1467] -> w1071
      tunnel: [w1466] -> w1070
      tunnel: [w1472] -> w655
      tunnel: [w1475] -> w885
      tunnel: [w1474] -> w886
      tunnel: [w1473] -> w858
      tunnel: w1073 -> [w1478]
      tunnel: w1072 -> [w1477]
      tunnel: w1071 -> [w1476]
      tunnel: w1070 -> [w1471]
      tunnel: [w1470] -> w719
      frame #0 {
        # "Write Data"
        n182 = To Long Integer(number="Max Number of Shots (Test intervals)") -> (32bit integer=w1465:i32)
        n183 = To Variant(anything=w1465) -> (Variant=w1466:variant)
      }
      frame #1 {
        # "Resolve To TC"
        n184 = call <userlib>:"Resolve To TC Type.vi"("Handle"=w1476, "TypHdl"=w1477, "WData"=w1471, "error in"=w1478) -> ("Handle"=w1474:u32, "TypHdl"=w1475:u32, "bHasMatched"=w1470:bool, "ADSWData"=w1473:variant, "error out"=w1472:errorcluster)  [unwired: 7 in]
      }
    }
    n185 = flat-sequence {
      tunnel: w846 -> [w1362]
      tunnel: w844 -> [w1363]
      tunnel: w845 -> [w1364]
      tunnel: [w1364] -> w857
      tunnel: [w1363] -> w856
      tunnel: [w1362] -> w855
      tunnel: [w1361] -> w854
      tunnel: w813 -> [w1359]
      tunnel: [w1367] -> w652
      tunnel: [w1370] -> w842
      tunnel: [w1369] -> w843
      tunnel: [w1368] -> w853
      tunnel: w857 -> [w1373]
      tunnel: w856 -> [w1372]
      tunnel: w855 -> [w1371]
      tunnel: w854 -> [w1366]
      tunnel: [w1365] -> w721
      frame #0 {
        # "Write Data"
        n186 = To Long Integer(number=w1359) -> (32bit integer=w1360:i32)
        n187 = To Variant(anything=w1360) -> (Variant=w1361:variant)
      }
      frame #1 {
        # "Resolve To TC"
        n188 = call <userlib>:"Resolve To TC Type.vi"("Handle"=w1371, "TypHdl"=w1372, "WData"=w1366, "error in"=w1373) -> ("Handle"=w1369:u32, "TypHdl"=w1370:u32, "bHasMatched"=w1365:bool, "ADSWData"=w1368:variant, "error out"=w1367:errorcluster)  [unwired: 7 in]
      }
    }
    n189 = flat-sequence {
      tunnel: w779 -> [w1342]
      tunnel: w778 -> [w1343]
      tunnel: w777 -> [w1340]
      tunnel: [w1340] -> w789
      tunnel: [w1343] -> w788
      tunnel: [w1342] -> w787
      tunnel: [w1341] -> w786
      tunnel: [w1346] -> w649
      tunnel: [w1349] -> w774
      tunnel: [w1348] -> w773
      tunnel: [w1347] -> w780
      tunnel: w789 -> [w1352]
      tunnel: w788 -> [w1351]
      tunnel: w787 -> [w1350]
      tunnel: w786 -> [w1345]
      tunnel: [w1344] -> w605
      frame #0 {
        # "Write Data"
        n190 = To Single Precision Float(number="Manual Charge Time (seconds)") -> (single precision float=w1338:sgl)
        n191 = To Variant(anything=w1338) -> (Variant=w1341:variant)
      }
      frame #1 {
        # "Resolve To TC"
        n192 = call <userlib>:"Resolve To TC Type.vi"("Handle"=w1350, "TypHdl"=w1351, "WData"=w1345, "error in"=w1352) -> ("Handle"=w1348:u32, "TypHdl"=w1349:u32, "bHasMatched"=w1344:bool, "ADSWData"=w1347:variant, "error out"=w1346:errorcluster)  [unwired: 7 in]
      }
    }
    n193 = flat-sequence {
      tunnel: w939 -> [w1527]
      tunnel: w938 -> [w1528]
      tunnel: w937 -> [w1529]
      tunnel: [w1529] -> w1089
      tunnel: [w1528] -> w1088
      tunnel: [w1527] -> w1087
      tunnel: [w1526] -> w1086
      tunnel: [w1532] -> w667
      tunnel: [w1535] -> w933
      tunnel: [w1534] -> w934
      tunnel: [w1533] -> w862
      tunnel: w1089 -> [w1538]
      tunnel: w1088 -> [w1537]
      tunnel: w1087 -> [w1536]
      tunnel: w1086 -> [w1531]
      tunnel: [w1530] -> w711
      frame #0 {
        # "Write Data"
        n194 = To Single Precision Float(number="Capacitance (uF)") -> (single precision float=w1525:sgl)
        n195 = To Variant(anything=w1525) -> (Variant=w1526:variant)
      }
      frame #1 {
        # "Resolve To TC"
        n196 = call <userlib>:"Resolve To TC Type.vi"("Handle"=w1536, "TypHdl"=w1537, "WData"=w1531, "error in"=w1538) -> ("Handle"=w1534:u32, "TypHdl"=w1535:u32, "bHasMatched"=w1530:bool, "ADSWData"=w1533:variant, "error out"=w1532:errorcluster)  [unwired: 7 in]
      }
    }
    n197 = flat-sequence {
      tunnel: w915 -> [w1497]
      tunnel: w914 -> [w1498]
      tunnel: w913 -> [w1499]
      tunnel: [w1499] -> w1081
      tunnel: [w1498] -> w1080
      tunnel: [w1497] -> w1079
      tunnel: [w1496] -> w1078
      tunnel: w772 -> [w1494]
      tunnel: [w1502] -> w661
      tunnel: [w1505] -> w909
      tunnel: [w1504] -> w910
      tunnel: [w1503] -> w860
      tunnel: w1081 -> [w1508]
      tunnel: w1080 -> [w1507]
      tunnel: w1079 -> [w1506]
      tunnel: w1078 -> [w1501]
      tunnel: [w1500] -> w715
      frame #0 {
        # "Write Data"
        n198 = To Long Integer(number=w1494) -> (32bit integer=w1495:i32)
        n199 = To Variant(anything=w1495) -> (Variant=w1496:variant)
      }
      frame #1 {
        # "Resolve To TC"
        n200 = call <userlib>:"Resolve To TC Type.vi"("Handle"=w1506, "TypHdl"=w1507, "WData"=w1501, "error in"=w1508) -> ("Handle"=w1504:u32, "TypHdl"=w1505:u32, "bHasMatched"=w1500:bool, "ADSWData"=w1503:variant, "error out"=w1502:errorcluster)  [unwired: 7 in]
      }
    }
    n201 = flat-sequence {
      tunnel: w947 -> [w1543]
      tunnel: [w1541] -> _
      tunnel: w945 -> [w1544]
      tunnel: [w1544] -> w1093
      tunnel: [w1541] -> w1092
      tunnel: [w1543] -> w1091
      tunnel: [w1542] -> w1090
      tunnel: w946 -> [w1541]
      tunnel: [w1547] -> w670
      tunnel: [w1550] -> w949
      tunnel: [w1549] -> w948
      tunnel: [w1548] -> w863
      tunnel: w1093 -> [w1553]
      tunnel: w1092 -> [w1552]
      tunnel: w1091 -> [w1551]
      tunnel: w1090 -> [w1546]
      tunnel: [w1545] -> w709
      frame #0 {
        # "Write Data"
        n202 = To Long Integer(number="Cycle Time (seconds)") -> (32bit integer=w1540:i32)
        n203 = To Variant(anything=w1540) -> (Variant=w1542:variant)
      }
      frame #1 {
        # "Resolve To TC"
        n204 = call <userlib>:"Resolve To TC Type.vi"("Handle"=w1551, "TypHdl"=w1552, "WData"=w1546, "error in"=w1553) -> ("Handle"=w1549:u32, "TypHdl"=w1550:u32, "bHasMatched"=w1545:bool, "ADSWData"=w1548:variant, "error out"=w1547:errorcluster)  [unwired: 7 in]
      }
    }
    n205 = flat-sequence {
      tunnel: w927 -> [w1512]
      tunnel: w926 -> [w1513]
      tunnel: w925 -> [w1514]
      tunnel: [w1514] -> w1085
      tunnel: [w1513] -> w1084
      tunnel: [w1512] -> w1083
      tunnel: [w1511] -> w1082
      tunnel: [w1517] -> w664
      tunnel: [w1520] -> w921
      tunnel: [w1519] -> w922
      tunnel: [w1518] -> w861
      tunnel: w1085 -> [w1523]
      tunnel: w1084 -> [w1522]
      tunnel: w1083 -> [w1521]
      tunnel: w1082 -> [w1516]
      tunnel: [w1515] -> w713
      frame #0 {
        # "Write Data"
        n206 = To Long Integer(number="Target Charge Volt (V) - Min 1500V - TEMPORARY LIMIT 12kV") -> (32bit integer=w1510:i32)
        n207 = To Variant(anything=w1510) -> (Variant=w1511:variant)
      }
      frame #1 {
        # "Resolve To TC"
        n208 = call <userlib>:"Resolve To TC Type.vi"("Handle"=w1521, "TypHdl"=w1522, "WData"=w1516, "error in"=w1523) -> ("Handle"=w1519:u32, "TypHdl"=w1520:u32, "bHasMatched"=w1515:bool, "ADSWData"=w1518:variant, "error out"=w1517:errorcluster)  [unwired: 7 in]
      }
    }
    n209 = flat-sequence {
      tunnel: w903 -> [w1482]
      tunnel: w902 -> [w1483]
      tunnel: w901 -> [w1484]
      tunnel: [w1484] -> w1077
      tunnel: [w1483] -> w1076
      tunnel: [w1482] -> w1075
      tunnel: [w1481] -> w1074
      tunnel: [w1487] -> w658
      tunnel: [w1490] -> w897
      tunnel: [w1489] -> w898
      tunnel: [w1488] -> w859
      tunnel: w1077 -> [w1493]
      tunnel: w1076 -> [w1492]
      tunnel: w1075 -> [w1491]
      tunnel: w1074 -> [w1486]
      tunnel: [w1485] -> w717
      frame #0 {
        # "Write Data"
        n210 = To Word Integer(number="Hold Time Before Shot (seconds)") -> (16bit integer=w1480:i16)
        n211 = To Variant(anything=w1480) -> (Variant=w1481:variant)
      }
      frame #1 {
        # "Resolve To TC"
        n212 = call <userlib>:"Resolve To TC Type.vi"("Handle"=w1491, "TypHdl"=w1492, "WData"=w1486, "error in"=w1493) -> ("Handle"=w1489:u32, "TypHdl"=w1490:u32, "bHasMatched"=w1485:bool, "ADSWData"=w1488:variant, "error out"=w1487:errorcluster)  [unwired: 7 in]
      }
    }
    n213 = flat-sequence {
      tunnel: w963 -> [w1377]
      tunnel: w962 -> [w1378]
      tunnel: w961 -> [w1379]
      tunnel: [w1379] -> w1049
      tunnel: [w1378] -> w1048
      tunnel: [w1377] -> w1047
      tunnel: [w1376] -> w1046
      tunnel: [w1382] -> w672
      tunnel: [w1385] -> w957
      tunnel: [w1384] -> w958
      tunnel: [w1383] -> w864
      tunnel: w1049 -> [w1388]
      tunnel: w1048 -> [w1387]
      tunnel: w1047 -> [w1386]
      tunnel: w1046 -> [w1381]
      tunnel: [w1380] -> w708
      frame #0 {
        # "Write Data"
        n214 = And(x="CLEAR FAULT", y="CLEAR FAULT") -> (x .and. y?=w1375:bool)
        n215 = To Variant(anything=w1375) -> (Variant=w1376:variant)
      }
      frame #1 {
        # "Resolve To TC"
        n216 = call <userlib>:"Resolve To TC Type.vi"("Handle"=w1386, "TypHdl"=w1387, "WData"=w1381, "error in"=w1388) -> ("Handle"=w1384:u32, "TypHdl"=w1385:u32, "bHasMatched"=w1380:bool, "ADSWData"=w1383:variant, "error out"=w1382:errorcluster)  [unwired: 7 in]
      }
    }
    n217 = flat-sequence {
      tunnel: w1011 -> [w1437]
      tunnel: w1010 -> [w1438]
      tunnel: w1009 -> [w1439]
      tunnel: [w1439] -> w1065
      tunnel: [w1438] -> w1064
      tunnel: [w1437] -> w1063
      tunnel: [w1436] -> w1062
      tunnel: [w1442] -> w684
      tunnel: [w1445] -> w1005
      tunnel: [w1444] -> w1006
      tunnel: [w1443] -> w868
      tunnel: w1065 -> [w1448]
      tunnel: w1064 -> [w1447]
      tunnel: w1063 -> [w1446]
      tunnel: w1062 -> [w1441]
      tunnel: [w1440] -> w700
      frame #0 {
        # "Write Data"
        n218 = And(x="Hold", y="Hold") -> (x .and. y?=w1435:bool)
        n219 = To Variant(anything=w1435) -> (Variant=w1436:variant)
      }
      frame #1 {
        # "Resolve To TC"
        n220 = call <userlib>:"Resolve To TC Type.vi"("Handle"=w1446, "TypHdl"=w1447, "WData"=w1441, "error in"=w1448) -> ("Handle"=w1444:u32, "TypHdl"=w1445:u32, "bHasMatched"=w1440:bool, "ADSWData"=w1443:variant, "error out"=w1442:errorcluster)  [unwired: 7 in]
      }
    }
    n221 = flat-sequence {
      tunnel: w987 -> [w1407]
      tunnel: w986 -> [w1408]
      tunnel: w985 -> [w1409]
      tunnel: [w1409] -> w1057
      tunnel: [w1408] -> w1056
      tunnel: [w1407] -> w1055
      tunnel: [w1406] -> w1054
      tunnel: [w1412] -> w678
      tunnel: [w1415] -> w981
      tunnel: [w1414] -> w982
      tunnel: [w1413] -> w866
      tunnel: w1057 -> [w1418]
      tunnel: w1056 -> [w1417]
      tunnel: w1055 -> [w1416]
      tunnel: w1054 -> [w1411]
      tunnel: [w1410] -> w704
      frame #0 {
        # "Write Data"
        n222 = And(x="Shot", y="Shot") -> (x .and. y?=w1405:bool)
        n223 = To Variant(anything=w1405) -> (Variant=w1406:variant)
      }
      frame #1 {
        # "Resolve To TC"
        n224 = call <userlib>:"Resolve To TC Type.vi"("Handle"=w1416, "TypHdl"=w1417, "WData"=w1411, "error in"=w1418) -> ("Handle"=w1414:u32, "TypHdl"=w1415:u32, "bHasMatched"=w1410:bool, "ADSWData"=w1413:variant, "error out"=w1412:errorcluster)  [unwired: 7 in]
      }
    }
    n225 = flat-sequence {
      tunnel: w1019 -> [w1453]
      tunnel: [w1449] -> _
      tunnel: w1017 -> [w1454]
      tunnel: [w1454] -> w1069
      tunnel: [w1449] -> w1068
      tunnel: [w1453] -> w1067
      tunnel: [w1452] -> w1066
      tunnel: w1018 -> [w1449]
      tunnel: [w1457] -> w687
      tunnel: [w1460] -> w1021
      tunnel: [w1459] -> w1020
      tunnel: [w1458] -> w869
      tunnel: w1069 -> [w1463]
      tunnel: w1068 -> [w1462]
      tunnel: w1067 -> [w1461]
      tunnel: w1066 -> [w1456]
      tunnel: [w1455] -> w698
      frame #0 {
        # "Write Data"
        n226 = And(x="Manual/Auto", y="Manual/Auto") -> (x .and. y?=w1451:bool)
        n227 = To Variant(anything=w1451) -> (Variant=w1452:variant)
      }
      frame #1 {
        # "Resolve To TC"
        n228 = call <userlib>:"Resolve To TC Type.vi"("Handle"=w1461, "TypHdl"=w1462, "WData"=w1456, "error in"=w1463) -> ("Handle"=w1459:u32, "TypHdl"=w1460:u32, "bHasMatched"=w1455:bool, "ADSWData"=w1458:variant, "error out"=w1457:errorcluster)  [unwired: 7 in]
      }
    }
    n229 = flat-sequence {
      tunnel: w999 -> [w1422]
      tunnel: w998 -> [w1423]
      tunnel: w997 -> [w1424]
      tunnel: [w1424] -> w1061
      tunnel: [w1423] -> w1060
      tunnel: [w1422] -> w1059
      tunnel: [w1421] -> w1058
      tunnel: [w1427] -> w681
      tunnel: [w1430] -> w993
      tunnel: [w1429] -> w994
      tunnel: [w1428] -> w867
      tunnel: w1061 -> [w1433]
      tunnel: w1060 -> [w1432]
      tunnel: w1059 -> [w1431]
      tunnel: w1058 -> [w1426]
      tunnel: [w1425] -> w702
      frame #0 {
        # "Write Data"
        n230 = And(x="Charge", y="Charge") -> (x .and. y?=w1420:bool)
        n231 = To Variant(anything=w1420) -> (Variant=w1421:variant)
      }
      frame #1 {
        # "Resolve To TC"
        n232 = call <userlib>:"Resolve To TC Type.vi"("Handle"=w1431, "TypHdl"=w1432, "WData"=w1426, "error in"=w1433) -> ("Handle"=w1429:u32, "TypHdl"=w1430:u32, "bHasMatched"=w1425:bool, "ADSWData"=w1428:variant, "error out"=w1427:errorcluster)  [unwired: 7 in]
      }
    }
    n233 = flat-sequence {
      tunnel: w975 -> [w1392]
      tunnel: w974 -> [w1393]
      tunnel: w973 -> [w1394]
      tunnel: [w1394] -> w1053
      tunnel: [w1393] -> w1052
      tunnel: [w1392] -> w1051
      tunnel: [w1391] -> w1050
      tunnel: [w1397] -> w675
      tunnel: [w1400] -> w969
      tunnel: [w1399] -> w970
      tunnel: [w1398] -> w865
      tunnel: w1053 -> [w1403]
      tunnel: w1052 -> [w1402]
      tunnel: w1051 -> [w1401]
      tunnel: w1050 -> [w1396]
      tunnel: [w1395] -> w706
      frame #0 {
        # "Write Data"
        n234 = And(x="HV Switch Mode", y="HV Switch Mode") -> (x .and. y?=w1390:bool)
        n235 = To Variant(anything=w1390) -> (Variant=w1391:variant)
      }
      frame #1 {
        # "Resolve To TC"
        n236 = call <userlib>:"Resolve To TC Type.vi"("Handle"=w1401, "TypHdl"=w1402, "WData"=w1396, "error in"=w1403) -> ("Handle"=w1399:u32, "TypHdl"=w1400:u32, "bHasMatched"=w1395:bool, "ADSWData"=w1398:variant, "error out"=w1397:errorcluster)  [unwired: 7 in]
      }
    }
    n237 = flat-sequence {
      tunnel: w1035 -> [w1323]
      tunnel: w1034 -> [w1324]
      tunnel: w1033 -> [w1325]
      tunnel: [w1325] -> w763
      tunnel: [w1324] -> w762
      tunnel: [w1323] -> w761
      tunnel: [w1322] -> w760
      tunnel: w763 -> [w1334]
      tunnel: w762 -> [w1333]
      tunnel: w761 -> [w1332]
      tunnel: w760 -> [w1327]
      tunnel: [w1328] -> w690
      tunnel: [w1331] -> w1029
      tunnel: [w1330] -> w1030
      tunnel: [w1329] -> w759
      tunnel: [w1326] -> w696
      frame #0 {
        # "Write Data"
        n238 = And(x="STOP", y="STOP") -> (x .and. y?=w1321:bool)
        n239 = To Variant(anything=w1321) -> (Variant=w1322:variant)
      }
      frame #1 {
        # "Resolve To TC"
        n240 = call <userlib>:"Resolve To TC Type.vi"("Handle"=w1332, "TypHdl"=w1333, "WData"=w1327, "error in"=w1334) -> ("Handle"=w1330:u32, "TypHdl"=w1331:u32, "bHasMatched"=w1326:bool, "ADSWData"=w1329:variant, "error out"=w1328:errorcluster)  [unwired: 7 in]
      }
    }
    n241 = flat-sequence {
      tunnel: w637 -> [w1270]
      tunnel: w636 -> [w1266]
      tunnel: w635 -> [w1271]
      tunnel: [w1271] -> w646
      tunnel: [w1266] -> w645
      tunnel: [w1270] -> w644
      tunnel: [w1269] -> w643
      tunnel: [w1274] -> w624
      tunnel: [w1277] -> w630
      tunnel: [w1276] -> w631
      tunnel: [w1275] -> w634
      tunnel: w646 -> [w1280]
      tunnel: w645 -> [w1279]
      tunnel: w644 -> [w1278]
      tunnel: w643 -> [w1273]
      tunnel: [w1272] -> w628
      frame #0 {
        # "Write Data"
        n242 = And(x="Reset Test Number", y="Reset Test Number") -> (x .and. y?=w1268:bool)
        n243 = To Variant(anything=w1268) -> (Variant=w1269:variant)
      }
      frame #1 {
        # "Resolve To TC"
        n244 = call <userlib>:"Resolve To TC Type.vi"("Handle"=w1278, "TypHdl"=w1279, "WData"=w1273, "error in"=w1280) -> ("Handle"=w1276:u32, "TypHdl"=w1277:u32, "bHasMatched"=w1272:bool, "ADSWData"=w1275:variant, "error out"=w1274:errorcluster)  [unwired: 7 in]
      }
    }
    n245 = flat-sequence {
      tunnel: w1045 -> [w1289]
      tunnel: w1044 -> [w1290]
      tunnel: w1041 -> [w1291]
      tunnel: [w1291] -> w758
      tunnel: [w1290] -> w757
      tunnel: [w1289] -> w756
      tunnel: [w1288] -> w755
      tunnel: [w1286] -> _
      tunnel: [w1286] -> w754
      tunnel: w771 -> [w1286]
      tunnel: w770 -> [w1285]
      tunnel: [w1285] -> w753
      tunnel: w769 -> [w1284]
      tunnel: [w1284] -> w752
      tunnel: w768 -> [w1283]
      tunnel: [w1283] -> w751
      tunnel: w767 -> [w1282]
      tunnel: [w1282] -> w750
      tunnel: ["START"] -> w545
      tunnel: w758 -> [w1305]
      tunnel: w757 -> [w1304]
      tunnel: w756 -> [w1303]
      tunnel: w755 -> [w1298]
      tunnel: [w1299] -> w749
      tunnel: [w1302] -> w748
      tunnel: [w1301] -> w747
      tunnel: [w1300] -> w746
      tunnel: [w1297] -> w745
      tunnel: w754 -> [w1296]
      tunnel: [w1296] -> w744
      tunnel: w753 -> [w1295]
      tunnel: [w1295] -> w743
      tunnel: w752 -> [w1294]
      tunnel: [w1294] -> w742
      tunnel: w751 -> [w1293]
      tunnel: [w1293] -> w741
      tunnel: [w1292] -> w740
      tunnel: w750 -> [w1292]
      tunnel: [w1316] -> w723
      tunnel: [w1317] -> w1043
      tunnel: [w1318] -> w1042
      tunnel: [w1319] -> w693
      tunnel: w749 -> [w1319]
      tunnel: w748 -> [w1318]
      tunnel: w747 -> [w1317]
      tunnel: w746 -> [w1308]
      tunnel: w745 -> [w1316]
      tunnel: w744 -> [w1315]
      tunnel: w743 -> [w1314]
      tunnel: w742 -> [w1313]
      tunnel: w741 -> [w1312]
      tunnel: w740 -> [w1311]
      tunnel: [w1310] -> w766
      tunnel: [w1309] -> w765
      tunnel: [w1307] -> w694
      tunnel: [w1306] -> w738
      frame #0 {
        # "Write Data"
        n246 = And(x="START", y="START") -> (x .and. y?=w1287:bool)
        n247 = To Variant(anything=w1287) -> (Variant=w1288:variant)
      }
      frame #1 {
        # "Resolve To TC"
        n248 = call <userlib>:"Resolve To TC Type.vi"("Handle"=w1303, "TypHdl"=w1304, "WData"=w1298, "error in"=w1305) -> ("Handle"=w1301:u32, "TypHdl"=w1302:u32, "bHasMatched"=w1297:bool, "ADSWData"=w1300:variant, "error out"=w1299:errorcluster)  [unwired: 7 in]
      }
      frame #2 {
        # "Write"
        n249 = call <userlib>:"Send Writer-Request.vi"("Handle"=w1315, "SymbolName"=w1314, "WriterMode"=w1313, "WriteHandle"=w1312, "error constant"=w1311, "ADS Write Data"=w1308) -> ("Handle"=w1310:u32, "WriteHandle"=w1309:u32, "Write status?"=w1306:bool, "error IO"=w1307:errorcluster)  [unwired: 5 in, 1 out]
      }
    }
    n250 = To Single Precision Float(number="Duty Cycle") -> (single precision float=w502:sgl)
    n251 = And(x="Voltage Held by PSU", y="Voltage Held by PSU") -> (x .and. y?=w488:bool)
    n252 = And(x="Current Control", y="Current Control") -> (x .and. y?=w509:bool)
    n253 = To Variant(anything=w502) -> (Variant=w506:variant)
    n254 = And(x="Dump", y="Dump") -> (x .and. y?=w518:bool)
    n255 = To Variant(anything=w488) -> (Variant=w486:variant)
    n256 = To Variant(anything=w509) -> (Variant=w507:variant)
    n257 = To Variant(anything=w518) -> (Variant=w519:variant)
    n258 = call-poly <userlib>:"Write TypeResolved.vi"("Handle"=w489, "SymbolName"=w490, "WData"=w486, "error constant"=w485) -> ("Write Status?"=w478:bool, "Has Matched?"=w479:bool, "error out"=w484:errorcluster)  [unwired: 8 in, 1 out]
    n259 = call-poly <userlib>:"Write TypeResolved.vi"("Handle"=w489, "SymbolName"=w510, "WData"=w506, "error constant"=w485) -> ("Write Status?"=w477:bool, "Has Matched?"=w480:bool, "error out"=w504:errorcluster)  [unwired: 8 in, 1 out]
    n260 = call-poly <userlib>:"Write TypeResolved.vi"("Handle"=w489, "SymbolName"=w511, "WData"=w507, "error constant"=w485) -> ("Write Status?"=w476:bool, "Has Matched?"=w481:bool, "error out"=w505:errorcluster)  [unwired: 8 in, 1 out]
    n261 = call <userlib>:"Send Writer-Request.vi"("Handle"=w1040, "SymbolName"=w1039, "WriterMode"=w1038, "WriteHandle"=w1037, "error constant"=w1036, "ADS Write Data"=w759) -> ("Handle"=w1032:u32, "WriteHandle"=w1031:u32, "Write status?"=w737:bool, "error IO"=w691:errorcluster)  [unwired: 5 in, 1 out]
    n262 = flat-sequence {
      tunnel: w884 -> [w1676]
      tunnel: w883 -> [w1674]
      tunnel: w882 -> [w1672]
      tunnel: [w1675] -> w1128
      tunnel: [w1673] -> w1127
      tunnel: [w1671] -> w1126
      tunnel: [w1670] -> w1125
      tunnel: [w1669] -> w1124
      tunnel: [w1668] -> w1123
      tunnel: [w1667] -> w1122
      tunnel: [w1666] -> w1121
      tunnel: [w1665] -> w1120
      tunnel: [w1664] -> w1119
      tunnel: [w1663] -> w1118
      tunnel: w880 -> [w1662]
      tunnel: w879 -> [w1661]
      tunnel: w878 -> [w1660]
      tunnel: w877 -> [w1659]
      tunnel: w876 -> [w1658]
      tunnel: w875 -> [w1657]
      tunnel: [w1656] -> w1117
      tunnel: [w1655] -> w1116
      tunnel: [w1654] -> w1115
      tunnel: [w1653] -> w1114
      tunnel: [w1652] -> w1113
      tunnel: [w1651] -> w1112
      tunnel: [w1650] -> w1111
      tunnel: [w1649] -> w1110
      tunnel: [w1648] -> w1109
      tunnel: [w1647] -> w1108
      tunnel: [w1646] -> w1107
      tunnel: [w1645] -> w1106
      tunnel: [w1644] -> w1105
      tunnel: [w1643] -> w1104
      tunnel: [w1642] -> w1103
      tunnel: [w1641] -> w1102
      tunnel: [w1640] -> w1101
      tunnel: [w1639] -> w1100
      tunnel: [w1638] -> w1099
      tunnel: [w1637] -> w1098
      tunnel: [w1636] -> w1097
      tunnel: [w1635] -> w1096
      tunnel: [w1634] -> w1095
      tunnel: [w1633] -> w1094
      tunnel: w840 -> [w1632]
      tunnel: [w1631] -> w839
      tunnel: [w1630] -> w838
      tunnel: [w1629] -> w837
      tunnel: [w1628] -> w836
      tunnel: [w1627] -> w835
      tunnel: w833 -> [w1557]
      tunnel: [w1626] -> w832
      tunnel: w830 -> [w1625]
      tunnel: [w1624] -> w829
      tunnel: [w1623] -> w828
      tunnel: [w1622] -> w827
      tunnel: w826 -> [w1621]
      tunnel: w825 -> [w1620]
      tunnel: [w1619] -> w824
      tunnel: [w1618] -> w823
      tunnel: [w1617] -> w822
      tunnel: [w1616] -> w821
      tunnel: [w1615] -> w820
      tunnel: [w1614] -> w819
      tunnel: [w1613] -> w818
      tunnel: [w1612] -> w817
      tunnel: w809 -> [w1611]
      tunnel: w808 -> [w1610]
      tunnel: w807 -> [w1609]
      tunnel: [w1608] -> w806
      tunnel: [w1607] -> w805
      tunnel: [w1606] -> w804
      tunnel: [w1605] -> w803
      tunnel: [w1604] -> w802
      tunnel: [w1603] -> w801
      tunnel: [w1602] -> w800
      tunnel: [w1601] -> w799
      tunnel: [w1600] -> w798
      tunnel: [w1599] -> w797
      tunnel: [w1598] -> w796
      tunnel: [w1597] -> w795
      tunnel: [w1558] -> _
      tunnel: w764 -> [w1558]
      tunnel: [w1596] -> w598
      tunnel: [w1595] -> w597
      tunnel: [w1594] -> w596
      tunnel: w595 -> [w1593]
      tunnel: [w1592] -> w590
      tunnel: w588 -> [w1591]
      tunnel: [w1590] -> w587
      tunnel: [w1589] -> w586
      tunnel: [w1588] -> w585
      tunnel: [w1587] -> w584
      tunnel: w583 -> [w1586]
      tunnel: w582 -> [w1585]
      tunnel: w581 -> [w1584]
      tunnel: [w1583] -> w580
      tunnel: [w1582] -> w579
      tunnel: [w1581] -> w577
      tunnel: [w1580] -> w575
      tunnel: [w1579] -> w574
      tunnel: [w1578] -> w573
      tunnel: [w1577] -> w572
      tunnel: [w1576] -> w569
      tunnel: w568 -> [w1575]
      tunnel: [w1574] -> w567
      tunnel: [w1573] -> w566
      tunnel: [w1572] -> w565
      tunnel: w543 -> [w1571]
      tunnel: w542 -> [w1570]
      tunnel: [w1569] -> w541
      tunnel: [w1568] -> w540
      tunnel: [w1567] -> w539
      tunnel: [w1566] -> w538
      tunnel: [w1565] -> w537
      tunnel: [w1564] -> w536
      tunnel: w535 -> [w1563]
      tunnel: [w1562] -> w534
      tunnel: [w1561] -> w533
      tunnel: [w1560] -> w532
      tunnel: w516 -> [w1559]
      tunnel: [w1556] -> w515
      tunnel: [w1555] -> w514
      tunnel: [w1554] -> w513
      tunnel: w1128 -> [w1853]
      tunnel: w1127 -> [w1866]
      tunnel: w1126 -> [_]
      tunnel: w1125 -> [w1852]
      tunnel: w1124 -> [w1851]
      tunnel: w1123 -> [w1867]
      tunnel: [w1768] -> w881
      tunnel: w1122 -> [w1865]
      tunnel: w1121 -> [w1868]
      tunnel: w1120 -> [w1870]
      tunnel: w1119 -> [w1828]
      tunnel: w1118 -> [_]
      tunnel: w1117 -> [w1848]
      tunnel: w1116 -> [w1863]
      tunnel: w1115 -> [w1861]
      tunnel: w1114 -> [w1859]
      tunnel: w1113 -> [w1857]
      tunnel: w1112 -> [w1855]
      tunnel: [w1781] -> w874
      tunnel: w1111 -> [w1847]
      tunnel: w1110 -> [w1846]
      tunnel: w1109 -> [w1845]
      tunnel: w1108 -> [w1844]
      tunnel: w1107 -> [w1843]
      tunnel: w1106 -> [w1842]
      tunnel: w1105 -> [_]
      tunnel: w1104 -> [w1841]
      tunnel: w1103 -> [_]
      tunnel: w1102 -> [w1840]
      tunnel: w1101 -> [_]
      tunnel: w1100 -> [w1839]
      tunnel: w1099 -> [_]
      tunnel: w1098 -> [w1838]
      tunnel: w1097 -> [_]
      tunnel: w1096 -> [w1837]
      tunnel: w1095 -> [_]
      tunnel: w1094 -> [w1836]
      tunnel: [w1783] -> w873
      tunnel: [w1785] -> w872
      tunnel: [w1787] -> w871
      tunnel: [w1789] -> w870
      tunnel: w839 -> [w1826]
      tunnel: w838 -> [w1825]
      tunnel: w837 -> [_]
      tunnel: w836 -> [w1751]
      tunnel: w835 -> [w1820]
      tunnel: [w1772] -> w834
      tunnel: w832 -> [w1824]
      tunnel: [w1770] -> w831
      tunnel: w829 -> [w1823]
      tunnel: w828 -> [w1821]
      tunnel: w827 -> [_]
      tunnel: w824 -> [w1817]
      tunnel: w823 -> [w1816]
      tunnel: w822 -> [w1813]
      tunnel: w821 -> [w1812]
      tunnel: w820 -> [w1811]
      tunnel: w819 -> [w1810]
      tunnel: w818 -> [_]
      tunnel: w817 -> [_]
      tunnel: [w1774] -> w816
      tunnel: [w1776] -> w815
      tunnel: [w1791] -> w812
      tunnel: [w1794] -> w811
      tunnel: [w1793] -> w810
      tunnel: w806 -> [w1808]
      tunnel: w805 -> [w1806]
      tunnel: w804 -> [w1804]
      tunnel: w803 -> [w1803]
      tunnel: w802 -> [w1802]
      tunnel: w801 -> [w1801]
      tunnel: w800 -> [w1800]
      tunnel: w799 -> [w1799]
      tunnel: w798 -> [w1798]
      tunnel: w797 -> [_]
      tunnel: w796 -> [_]
      tunnel: w795 -> [_]
      tunnel: [w1779] -> w794
      tunnel: [w1777] -> w793
      tunnel: [w1766] -> w792
      tunnel: [w1767] -> w791
      tunnel: [w1757] -> w647
      tunnel: [w1759] -> w599
      tunnel: w598 -> [w1763]
      tunnel: w597 -> [w1762]
      tunnel: w596 -> [_]
      tunnel: [w1760] -> w594
      tunnel: w590 -> [w1754]
      tunnel: w587 -> [w1749]
      tunnel: w586 -> [w1746]
      tunnel: w585 -> [w1744]
      tunnel: w584 -> [w1727]
      tunnel: w580 -> [w1743]
      tunnel: w579 -> [w1742]
      tunnel: [w1741] -> w578
      tunnel: w577 -> [w1740]
      tunnel: [w1739] -> w576
      tunnel: w575 -> [w1738]
      tunnel: w574 -> [w1737]
      tunnel: w573 -> [w1736]
      tunnel: w572 -> [w1735]
      tunnel: [w1734] -> w571
      tunnel: [w1733] -> w570
      tunnel: w569 -> [w1732]
      tunnel: [w1731] -> w552
      tunnel: [w1730] -> w550
      tunnel: [w1729] -> w560
      tunnel: w567 -> [w1721]
      tunnel: w566 -> [w1725]
      tunnel: w565 -> [w1724]
      tunnel: [w1723] -> w564
      tunnel: w541 -> [w1716]
      tunnel: w540 -> [w1719]
      tunnel: w539 -> [w1718]
      tunnel: w538 -> [w1717]
      tunnel: w537 -> [w1711]
      tunnel: w536 -> [w1714]
      tunnel: w534 -> [w1695]
      tunnel: w533 -> [w1710]
      tunnel: w532 -> [w1709]
      tunnel: [w1702] -> w531
      tunnel: [w1701] -> w530
      tunnel: [w1700] -> w529
      tunnel: [w1699] -> w528
      tunnel: w515 -> [w1696]
      tunnel: w514 -> [w1693]
      tunnel: w513 -> [w1692]
      tunnel: [w1691] -> w512
      frame #0 {
        # "Read and Resolve Data."
        # "Read/Resolve Symbol N"
        # "Read Data and Resolve Type"
        n263 = call-poly <userlib>:"Read TypeResolved.vi"("Handle"=w1558, "SymbolName"=w1620, "error constant"=w1557) -> ("Handle"=w1613:u32, "Read Status?"=w1618:bool, "RData"=w1614:variant, "error out"=w1617:errorcluster)  [unwired: 9 in]
        n264 = call-poly <userlib>:"Read TypeResolved.vi"("Handle"=w1558, "SymbolName"=w1621, "error constant"=w1557) -> ("Handle"=w1612:u32, "Read Status?"=w1619:bool, "RData"=w1615:variant, "error out"=w1616:errorcluster)  [unwired: 9 in]
        n265 = call-poly <userlib>:"Read TypeResolved.vi"("Handle"=w1558, "SymbolName"=w1674, "error constant"=w1557) -> ("Handle"=w1664:u32, "Read Status?"=w1666:bool, "RData"=w1670:variant, "error out"=w1675:errorcluster)  [unwired: 9 in]
        n266 = call-poly <userlib>:"Read TypeResolved.vi"("Handle"=w1558, "SymbolName"=w1625, "error constant"=w1557) -> ("Handle"=w1622:u32, "Read Status?"=w1624:bool, "RData"=w1623:variant, "error out"=w1627:errorcluster)  [unwired: 9 in]
        n267 = call-poly <userlib>:"Read TypeResolved.vi"("Handle"=w1558, "SymbolName"=w1676, "error constant"=w1557) -> ("Handle"=w1663:u32, "Read Status?"=w1665:bool, "RData"=w1669:variant, "error out"=w1626:errorcluster)  [unwired: 9 in]
        n268 = call-poly <userlib>:"Read TypeResolved.vi"("Handle"=w1558, "SymbolName"=w1672) -> ("Handle"=w1671:u32, "Read Status?"=w1667:bool, "RData"=w1668:variant, "error out"=w1673:errorcluster)  [unwired: 10 in]
        n269 = call-poly <userlib>:"Read TypeResolved.vi"("Handle"=w1558, "SymbolName"=w1662, "error constant"=w1557) -> ("Handle"=w1644:u32, "Read Status?"=w1651:bool, "RData"=w1643:variant, "error out"=w1650:errorcluster)  [unwired: 9 in]
        n270 = call-poly <userlib>:"Read TypeResolved.vi"("Handle"=w1558, "SymbolName"=w1563, "error constant"=w1557) -> ("Read Status?"=w1562:bool, "RData"=w1561:variant, "error out"=w1560:errorcluster)  [unwired: 9 in, 1 out]
        n271 = call-poly <userlib>:"Read TypeResolved.vi"("Handle"=w1558, "SymbolName"=w1559, "error constant"=w1557) -> ("Read Status?"=w1556:bool, "RData"=w1554:variant, "error out"=w1555:errorcluster)  [unwired: 9 in, 1 out]
        n272 = call-poly <userlib>:"Read TypeResolved.vi"("Handle"=w1558, "SymbolName"=w1660, "error constant"=w1557) -> ("Handle"=w1640:u32, "Read Status?"=w1653:bool, "RData"=w1639:variant, "error out"=w1648:errorcluster)  [unwired: 9 in]
        n273 = call-poly <userlib>:"Read TypeResolved.vi"("Handle"=w1558, "SymbolName"=w1658, "error constant"=w1557) -> ("Handle"=w1636:u32, "Read Status?"=w1655:bool, "RData"=w1635:variant, "error out"=w1646:errorcluster)  [unwired: 9 in]
        n274 = call-poly <userlib>:"Read TypeResolved.vi"("Handle"=w1558, "SymbolName"=w1575, "error constant"=w1557) -> ("Read Status?"=w1574:bool, "RData"=w1573:variant, "error out"=w1572:errorcluster)  [unwired: 9 in, 1 out]
        n275 = call-poly <userlib>:"Read TypeResolved.vi"("Handle"=w1558, "SymbolName"=w1571, "error constant"=w1557) -> ("Read Status?"=w1569:bool, "RData"=w1568:variant, "error out"=w1567:errorcluster)  [unwired: 9 in, 1 out]
        n276 = call-poly <userlib>:"Read TypeResolved.vi"("Handle"=w1558, "SymbolName"=w1570, "error constant"=w1557) -> ("Read Status?"=w1565:bool, "RData"=w1564:variant, "error out"=w1566:errorcluster)  [unwired: 9 in, 1 out]
        n277 = call-poly <userlib>:"Read TypeResolved.vi"("Handle"=w1558, "SymbolName"=w1661, "error constant"=w1557) -> ("Handle"=w1642:u32, "Read Status?"=w1652:bool, "RData"=w1641:variant, "error out"=w1649:errorcluster)  [unwired: 9 in]
        n278 = call-poly <userlib>:"Read TypeResolved.vi"("Handle"=w1558, "SymbolName"=w1659, "error constant"=w1557) -> ("Handle"=w1638:u32, "Read Status?"=w1654:bool, "RData"=w1637:variant, "error out"=w1647:errorcluster)  [unwired: 9 in]
        n279 = call-poly <userlib>:"Read TypeResolved.vi"("Handle"=w1558, "SymbolName"=w1657, "error constant"=w1557) -> ("Handle"=w1634:u32, "Read Status?"=w1656:bool, "RData"=w1633:variant, "error out"=w1645:errorcluster)  [unwired: 9 in]
        n280 = call-poly <userlib>:"Read TypeResolved.vi"("Handle"=w1558, "SymbolName"=w1632, "error constant"=w1557) -> ("Handle"=w1629:u32, "Read Status?"=w1628:bool, "RData"=w1631:variant, "error out"=w1630:errorcluster)  [unwired: 9 in]
        n281 = call-poly <userlib>:"Read TypeResolved.vi"("Handle"=w1558, "SymbolName"=w1591, "error constant"=w1557) -> ("Read Status?"=w1590:bool, "RData"=w1583:variant, "error out"=w1582:errorcluster)  [unwired: 9 in, 1 out]
        n282 = call-poly <userlib>:"Read TypeResolved.vi"("Handle"=w1558, "SymbolName"=w1586, "error constant"=w1557) -> ("Read Status?"=w1589:bool, "RData"=w1576:variant, "error out"=w1581:errorcluster)  [unwired: 9 in, 1 out]
        n283 = call-poly <userlib>:"Read TypeResolved.vi"("Handle"=w1558, "SymbolName"=w1584, "error constant"=w1557) -> ("Read Status?"=w1587:bool, "RData"=w1577:variant, "error out"=w1578:errorcluster)  [unwired: 9 in, 1 out]
        n284 = call-poly <userlib>:"Read TypeResolved.vi"("Handle"=w1558, "SymbolName"=w1585, "error constant"=w1557) -> ("Read Status?"=w1588:bool, "RData"=w1579:variant, "error out"=w1580:errorcluster)  [unwired: 9 in, 1 out]
        n285 = call-poly <userlib>:"Read TypeResolved.vi"("Handle"=w1558, "SymbolName"=w1611, "error constant"=w1557) -> ("Handle"=w1599:u32, "Read Status?"=w1608:bool, "RData"=w1604:variant, "error out"=w1600:errorcluster)  [unwired: 9 in]
        n286 = call-poly <userlib>:"Read TypeResolved.vi"("Handle"=w1558, "SymbolName"=w1610, "error constant"=w1557) -> ("Handle"=w1598:u32, "Read Status?"=w1607:bool, "RData"=w1605:variant, "error out"=w1601:errorcluster)  [unwired: 9 in]
        n287 = call-poly <userlib>:"Read TypeResolved.vi"("Handle"=w1558, "SymbolName"=w1593, "error constant"=w1557) -> ("Handle"=w1594:u32, "Read Status?"=w1592:bool, "RData"=w1596:variant, "error out"=w1595:errorcluster)  [unwired: 9 in]
        n288 = call-poly <userlib>:"Read TypeResolved.vi"("Handle"=w1558, "SymbolName"=w1609, "error constant"=w1557) -> ("Handle"=w1597:u32, "Read Status?"=w1606:bool, "RData"=w1603:variant, "error out"=w1602:errorcluster)  [unwired: 9 in]
      }
      frame #1 {
        # "Cast Symbol N to LabVIEW Type"
        # "Variant To Data"
        n289 = And(x=w1695, y=w1696) -> (x .and. y?=w1694:bool)
        n290 = And(x=w1711, y=w1694) -> (x .and. y?=w1712:bool)
        n291 = And(x=w1716, y=w1712) -> (x .and. y?=w1715:bool)
        n292 = And(x=w1721, y=w1715) -> (x .and. y?=w1720:bool)
        n293 = And(x=w1727, y=w1720) -> (x .and. y?=w1726:bool)
        n294 = And(x=w1744, y=w1726) -> (x .and. y?=w1745:bool)
        n295 = And(x=w1746, y=w1745) -> (x .and. y?=w1747:bool)
        n296 = And(x=w1749, y=w1747) -> (x .and. y?=w1748:bool)
        n297 = And(x=w1751, y=w1748) -> (x .and. y?=w1750:bool)
        n298 = And(x=w1848, y=w1750) -> (x .and. y?=w1864:bool)
        n299 = And(x=w1863, y=w1864) -> (x .and. y?=w1862:bool)
        n300 = And(x=w1861, y=w1862) -> (x .and. y?=w1860:bool)
        n301 = And(x=w1859, y=w1860) -> (x .and. y?=w1858:bool)
        n302 = And(x=w1857, y=w1858) -> (x .and. y?=w1856:bool)
        n303 = And(x=w1855, y=w1856) -> (x .and. y?=w1854:bool)
        n304 = And(x=w1865, y=w1854) -> (x .and. y?=w1809:bool)
        n305 = And(x=w1808, y=w1809) -> (x .and. y?=w1807:bool)
        n306 = And(x=w1806, y=w1807) -> (x .and. y?=w1805:bool)
        n307 = And(x=w1804, y=w1805) -> (x .and. y?=w1753:bool)
        n308 = And(x=w1754, y=w1753) -> (x .and. y?=w1752:bool)
        n309 = And(x=w1816, y=w1752) -> (x .and. y?=w1815:bool)
        n310 = And(x=w1817, y=w1815) -> (x .and. y?=w1814:bool)
        n311 = And(x=w1823, y=w1814) -> (x .and. y?=w1822:bool)
        n312 = And(x=w1870, y=w1822) -> (x .and. y?=w1869:bool)
        n313 = Variant To Data(error in=w1762, Variant=w1763) -> (data=→"Cap 1 Voltage (HVPS)":i16, error out=w1760:errorcluster)  [unwired: 1 in]
        n314 = Variant To Data(error in=w1847, Variant=w1841) -> (data=→"Discharge Fault":bool, error out=w1783:errorcluster)  [unwired: 1 in]
        n315 = Variant To Data(error in=w1866, Variant=w1867) -> (data=→"Charge Fault":bool, error out=w1781:errorcluster)  [unwired: 1 in]
        n316 = Variant To Data(error in=w1845, Variant=w1839) -> (data=→"Cap 1 Temp\nExceeded Fault":bool, error out=w1787:errorcluster)  [unwired: 1 in]
        n317 = And(x=w1868, y=w1869) -> (x .and. y?=→"Read Status":bool)
        n318 = Variant To Data(error in=w1846, Variant=w1840) -> (data=→"Hold Fault":bool, error out=w1785:errorcluster)  [unwired: 1 in]
        n319 = Variant To Data(error in=w1800, Variant=w1801) -> (data=→"Load Temperature":i16, error out=w1766:errorcluster)  [unwired: 1 in]
        n320 = Variant To Data(error in=w1844, Variant=w1838) -> (data=→"Ambient Temp\nExceeded Fault":bool, error out=w1789:errorcluster)  [unwired: 1 in]
        n321 = Variant To Data(error in=w1843, Variant=w1837) -> (data=→"PSU Fault":bool, error out=w1791:errorcluster)  [unwired: 1 in]
        n322 = Variant To Data(error in=w1842, Variant=w1836) -> (data=→"Control Sys Fault":bool, error out=w1793:errorcluster)  [unwired: 1 in]
        n323 = Variant To Data(error in=w1825, Variant=w1826) -> (data=→"test Running":bool, error out=w1794:errorcluster)  [unwired: 1 in]
        n324 = Variant To Data(error in=w1798, Variant=w1802) -> (data=→"Ambient Temp":i16, error out=w1779:errorcluster)  [unwired: 1 in]
        n325 = Variant To Data(error in=w1736, Variant=w1735) -> (data=w1729:bool, error out=w1733:errorcluster)  [unwired: 1 in]
        "Soft Exception" <- w1729
        n326 = Variant To Data(error in=w1724, Variant=w1725) -> (data=w1722:bool, error out=w1702:errorcluster)  [unwired: 1 in]
        "EOC" <- w1722
        n327 = Variant To Data(error in=w1799, Variant=w1803) -> (data=→"Soft Dump Temp":i16, error out=w1777:errorcluster)  [unwired: 1 in]
        n328 = Variant To Data(error in=w1742, Variant=w1743) -> (data=w1723:bool, error out=w1741:errorcluster)  [unwired: 1 in]
        "Softdump FB Fault" <- w1723
        n329 = Variant To Data(error in=w1738, Variant=w1737) -> (data=w1730:bool, error out=w1734:errorcluster)  [unwired: 1 in]
        "PSU HV FB Fault" <- w1730
        n330 = Variant To Data(error in=w1718, Variant=w1719) -> (data=w1688:bool, error out=w1701:errorcluster)  [unwired: 1 in]
        "SCR Ready" <- w1688
        n331 = Variant To Data(error in=w1717, Variant=w1714) -> (data=→"Maximum Test Number Reached":bool, error out=w1700:errorcluster)  [unwired: 1 in]
        n332 = Variant To Data(error in=w1740, Variant=w1732) -> (data=w1731:bool, error out=w1739:errorcluster)  [unwired: 1 in]
        "Charge FB Fault" <- w1731
        n333 = Variant To Data(error in=w1693, Variant=w1692) -> (data=w1689:bool, error out=w1691:errorcluster)  [unwired: 1 in]
        "Scope Trig" <- w1689
        n334 = Variant To Data(error in=w1820, type=2, Variant=w1821) -> (data=w1690:i32, error out=w1772:errorcluster)
        "Process Step" <- w1690
        n335 = Variant To Data(error in=w1813, Variant=w1810) -> (data=→"Cap 1 Temperature":i16, error out=w1776:errorcluster)  [unwired: 1 in]
        n336 = Variant To Data(error in=w1812, Variant=w1811) -> (data=w1708:i16, error out=w1774:errorcluster)  [unwired: 1 in]
        "Cap 1 Voltage" <- w1708
        n337 = Variant To Data(error in=w1709, Variant=w1710) -> (data=w1698:i16, error out=w1699:errorcluster)  [unwired: 1 in]
        "Expected Voltage" <- w1698
        n338 = Variant To Data(error in=w1853, Variant=w1852) -> (data=→"Estimated Charge Time (seconds)":sgl, error out=w1768:errorcluster)  [unwired: 1 in]
        n339 = To Double Precision Float(number=w1708) -> (double precision float=→"Waveform Chart - Capacitor Voltage (Probe, abs(Volts))":dbl)
        n340 = Variant To Data(error in=w1824, Variant=w1851) -> (data=→"Shot Number":i32, error out=w1770:errorcluster)  [unwired: 1 in]
        n341 = case shown="True" "Log Temperature Data" {
          tunnel: [errorcluster {"status"=FALSE, "code"=0, "source"=""} ("error out") w1880] -> w1759
          frame False {
          }
          frame True {
            n342 = local read "Cap 1 Temperature"() -> (w1881:i16)
            n343 = local read "test Running"() -> (w1879:bool)
            n344 = call "Write To Measurement File2"("Signals"=w1881, "Enable"=w1879, "Filename"="Capacitor Temperature Data Log File Path (.xlsx)") -> ("error out"=w1880:errorcluster)  [unwired: 14 in, 2 out]
          }
        }
        n345 = case shown="5" w1690 {
          tunnel: ["Charge" "Current Controlled Charge" "Hold - Ready for Shot" "Hold - Cap Open Circuited" "Shot" "Wait" "Dump" "Error" "Wait"] -> w1819
          tunnel: [TRUE TRUE TRUE TRUE TRUE TRUE FALSE FALSE FALSE] -> w1686
          tunnel: [FALSE ("Reset") FALSE ("Reset") FALSE ("Reset") FALSE ("Reset") TRUE ("Reset") FALSE ("Reset") FALSE ("Reset") TRUE ("Reset") FALSE ("Reset")] -> _
          frame 1 {
          }
          frame 6 {
          }
          frame 2 {
          }
          frame 7 {
          }
          frame 3 {
          }
          frame 4 {
          }
          frame 5 {
          }
          frame 999 {
          }
          frame 0, Default {
          }
        }
        "Test State" <- w1819
        n346 = local write "Scope Trig"(w1689) -> ()
        n347 = local read "Cap 1 Voltage"() -> (w1678:i16)
        n348 = case shown="True" "Log Capacitor Voltage" {
          tunnel: [errorcluster {"status"=FALSE, "code"=0, "source"=""} ("error out") w1877] -> w1757
          tunnel: w1708 -> [_ w1876]
          tunnel: w1686 -> [_ w1875]
          frame False {
          }
          frame True {
            n349 = local read "test Running"() -> (w1872:bool)
            n350 = And(x=w1875, y=w1872) -> (x .and. y?=w1873:bool)
            n351 = call "Write To Measurement File"("Signals"=w1876, "Enable"=w1873, "Filename"="Capacitor Voltage Data Log File Path (.xlsx)") -> ("error out"=w1877:errorcluster)  [unwired: 14 in, 2 out]
          }
        }
        n352 = Not(x=w1722) -> (.not. x?=w1706:bool)
        n353 = To Double Precision Float(number=w1678) -> (double precision float=w1704:dbl)
        n354 = To Double Precision Float(number=w1698) -> (double precision float=w1697:dbl)
        n355 = Boolean To (0,1)(Boolean=w1706) -> (0, 1=→"EOC":i16)
        n356 = Or(x=w1793, y=w1794) -> (x .or. y?=w1792:bool)
        n357 = Or(x=w1791, y=w1792) -> (x .or. y?=w1790:bool)
        n358 = Or(x=w1789, y=w1790) -> (x .or. y?=w1788:bool)
        n359 = Or(x=w1787, y=w1788) -> (x .or. y?=w1786:bool)
        n360 = Or(x=w1785, y=w1786) -> (x .or. y?=w1784:bool)
        n361 = Or(x=w1783, y=w1784) -> (x .or. y?=w1782:bool)
        n362 = Or(x=w1781, y=w1782) -> (x .or. y?=w1780:bool)
        n363 = Or(x=w1779, y=w1780) -> (x .or. y?=w1778:bool)
        n364 = Or(x=w1777, y=w1778) -> (x .or. y?=w1765:bool)
        n365 = Or(x=w1766, y=w1765) -> (x .or. y?=w1758:bool)
        n366 = Boolean To (0,1)(Boolean=w1688) -> (0, 1=→"SCR FB":i16)
        n367 = Bundle(w1704, w1697) -> (→"Capacitor Voltage":cluster{dbl, dbl})  [unwired: 1 in]
        n368 = local read "Scope Trig"() -> (w1681:bool)
        n369 = local write "Process Step"(w1690) -> ()
        n370 = Not(x=w1681) -> (.not. x?=w1680:bool)
        n371 = local read "Cycle Time (seconds)"() -> (w1684:i32)
        n372 = call "Elapsed Time"("Time Target (s)"=w1684, "Reset"=w1680) -> ("Elapsed Time Text"=w1683:string)  [unwired: 10 in, 7 out]
        n373 = String Subset(string=w1683, offset (0)=2) -> (substring=→"Time Since Last Shot":string)  [unwired: 1 in]
        n374 = Or(x=w1759, y=w1758) -> (x .or. y?=w1756:bool)
        n375 = Or(x=w1757, y=w1756) -> (x .or. y?=w1755:bool)
        n376 = Or(x=w1776, y=w1755) -> (x .or. y?=w1775:bool)
        n377 = Or(x=w1774, y=w1775) -> (x .or. y?=w1773:bool)
        n378 = Or(x=w1772, y=w1773) -> (x .or. y?=w1771:bool)
        n379 = Or(x=w1770, y=w1771) -> (x .or. y?=w1769:bool)
        n380 = Or(x=w1768, y=w1769) -> (x .or. y?=w1767:bool)
        "Internal TwinCAT Handle ID Maps" <- w1828
      }
    }
    n381 = call-poly <userlib>:"Write TypeResolved.vi"("Handle"=w489, "SymbolName"=w527, "WData"=w519, "error constant"=w526) -> ("Handle"=w520:u32, "Write Status?"=w475:bool, "Has Matched?"=w483:bool, "error out"=w521:errorcluster)  [unwired: 8 in]
    n382 = call <userlib>:"Send Writer-Request.vi"("Handle"=w785, "SymbolName"=w784, "WriterMode"=w783, "WriteHandle"=w781, "error constant"=w782, "ADS Write Data"=w780) -> ("Handle"=w776:u32, "WriteHandle"=w775:u32, "Write status?"=w602:bool, "error IO"=w650:errorcluster)  [unwired: 5 in, 1 out]
    n383 = call <userlib>:"Send Writer-Request.vi"("Handle"=w618, "SymbolName"=w617, "WriterMode"=w616, "WriteHandle"=w615, "error constant"=w614, "ADS Write Data"=w610) -> ("Handle"=w609:u32, "WriteHandle"=w606:u32, "Write status?"=w525:bool, "error IO"=w601:errorcluster)  [unwired: 5 in, 1 out]
    n384 = call <userlib>:"Send Writer-Request.vi"("Handle"=w956, "SymbolName"=w955, "WriterMode"=w954, "WriteHandle"=w952, "error constant"=w953, "ADS Write Data"=w863) -> ("Handle"=w951:u32, "WriteHandle"=w950:u32, "Write status?"=w501:bool, "error IO"=w671:errorcluster)  [unwired: 5 in, 1 out]
    n385 = call <userlib>:"Send Writer-Request.vi"("Handle"=w896, "SymbolName"=w895, "WriterMode"=w894, "WriteHandle"=w893, "error constant"=w892, "ADS Write Data"=w858) -> ("Handle"=w888:u32, "WriteHandle"=w887:u32, "Write status?"=w496:bool, "error IO"=w656:errorcluster)  [unwired: 5 in, 1 out]
    n386 = call <userlib>:"Send Writer-Request.vi"("Handle"=w852, "SymbolName"=w851, "WriterMode"=w850, "WriteHandle"=w841, "error constant"=w849, "ADS Write Data"=w853) -> ("Handle"=w848:u32, "WriteHandle"=w847:u32, "Write status?"=w495:bool, "error IO"=w653:errorcluster)  [unwired: 5 in, 1 out]
    n387 = call <userlib>:"Send Writer-Request.vi"("Handle"=w944, "SymbolName"=w943, "WriterMode"=w942, "WriteHandle"=w941, "error constant"=w940, "ADS Write Data"=w862) -> ("Handle"=w936:u32, "WriteHandle"=w935:u32, "Write status?"=w500:bool, "error IO"=w668:errorcluster)  [unwired: 5 in, 1 out]
    n388 = call <userlib>:"Send Writer-Request.vi"("Handle"=w920, "SymbolName"=w919, "WriterMode"=w918, "WriteHandle"=w917, "error constant"=w916, "ADS Write Data"=w860) -> ("Handle"=w912:u32, "WriteHandle"=w911:u32, "Write status?"=w498:bool, "error IO"=w662:errorcluster)  [unwired: 5 in, 1 out]
    n389 = call <userlib>:"Send Writer-Request.vi"("Handle"=w932, "SymbolName"=w931, "WriterMode"=w930, "WriteHandle"=w929, "error constant"=w928, "ADS Write Data"=w861) -> ("Handle"=w924:u32, "WriteHandle"=w923:u32, "Write status?"=w499:bool, "error IO"=w665:errorcluster)  [unwired: 5 in, 1 out]
    n390 = call <userlib>:"Send Writer-Request.vi"("Handle"=w908, "SymbolName"=w907, "WriterMode"=w906, "WriteHandle"=w905, "error constant"=w904, "ADS Write Data"=w859) -> ("Handle"=w900:u32, "WriteHandle"=w899:u32, "Write status?"=w497:bool, "error IO"=w659:errorcluster)  [unwired: 5 in, 1 out]
    n391 = call <userlib>:"Send Writer-Request.vi"("Handle"=w1028, "SymbolName"=w1027, "WriterMode"=w1026, "WriteHandle"=w1024, "error constant"=w1025, "ADS Write Data"=w869) -> ("Handle"=w1023:u32, "WriteHandle"=w1022:u32, "Write status?"=w725:bool, "error IO"=w688:errorcluster)  [unwired: 5 in, 1 out]
    n392 = call <userlib>:"Send Writer-Request.vi"("Handle"=w968, "SymbolName"=w967, "WriterMode"=w966, "WriteHandle"=w965, "error constant"=w964, "ADS Write Data"=w864) -> ("Handle"=w960:u32, "WriteHandle"=w959:u32, "Write status?"=w735:bool, "error IO"=w673:errorcluster)  [unwired: 5 in, 1 out]
    n393 = call <userlib>:"Send Writer-Request.vi"("Handle"=w1016, "SymbolName"=w1015, "WriterMode"=w1014, "WriteHandle"=w1013, "error constant"=w1012, "ADS Write Data"=w868) -> ("Handle"=w1008:u32, "WriteHandle"=w1007:u32, "Write status?"=w727:bool, "error IO"=w685:errorcluster)  [unwired: 5 in, 1 out]
    n394 = call <userlib>:"Send Writer-Request.vi"("Handle"=w992, "SymbolName"=w991, "WriterMode"=w990, "WriteHandle"=w989, "error constant"=w988, "ADS Write Data"=w866) -> ("Handle"=w984:u32, "WriteHandle"=w983:u32, "Write status?"=w731:bool, "error IO"=w679:errorcluster)  [unwired: 5 in, 1 out]
    n395 = call <userlib>:"Send Writer-Request.vi"("Handle"=w1004, "SymbolName"=w1003, "WriterMode"=w1002, "WriteHandle"=w1001, "error constant"=w1000, "ADS Write Data"=w867) -> ("Handle"=w996:u32, "WriteHandle"=w995:u32, "Write status?"=w729:bool, "error IO"=w682:errorcluster)  [unwired: 5 in, 1 out]
    n396 = call <userlib>:"Send Writer-Request.vi"("Handle"=w980, "SymbolName"=w979, "WriterMode"=w978, "WriteHandle"=w977, "error constant"=w976, "ADS Write Data"=w865) -> ("Handle"=w972:u32, "WriteHandle"=w971:u32, "Write status?"=w733:bool, "error IO"=w676:errorcluster)  [unwired: 5 in, 1 out]
    n397 = call <userlib>:"Send Writer-Request.vi"("Handle"=w642, "SymbolName"=w641, "WriterMode"=w640, "WriteHandle"=w639, "error constant"=w638, "ADS Write Data"=w634) -> ("Handle"=w633:u32, "WriteHandle"=w632:u32, "Write status?"=w626:bool, "error IO"=w625:errorcluster)  [unwired: 5 in, 1 out]
    n398 = Compound Arithmetic op=AND(w483, w481, w480, w479) -> (w482:bool)
    n399 = And(x=w523, y=w482) -> (x .and. y?=w522:bool)
    n400 = And(x=w605, y=w522) -> (x .and. y?=w604:bool)
    n401 = And(x=w721, y=w604) -> (x .and. y?=w720:bool)
    n402 = And(x=w719, y=w720) -> (x .and. y?=w718:bool)
    n403 = And(x=w717, y=w718) -> (x .and. y?=w716:bool)
    n404 = And(x=w715, y=w716) -> (x .and. y?=w714:bool)
    n405 = And(x=w713, y=w714) -> (x .and. y?=w712:bool)
    n406 = And(x=w711, y=w712) -> (x .and. y?=w710:bool)
    n407 = And(x=w709, y=w710) -> (x .and. y?=w592:bool)
    n408 = And(x=w628, y=w592) -> (x .and. y?=w629:bool)
    n409 = And(x=w708, y=w629) -> (x .and. y?=w707:bool)
    n410 = And(x=w706, y=w707) -> (x .and. y?=w705:bool)
    n411 = And(x=w704, y=w705) -> (x .and. y?=w703:bool)
    n412 = And(x=w702, y=w703) -> (x .and. y?=w701:bool)
    n413 = And(x=w700, y=w701) -> (x .and. y?=w699:bool)
    n414 = And(x=w698, y=w699) -> (x .and. y?=w697:bool)
    n415 = And(x=w696, y=w697) -> (x .and. y?=w695:bool)
    n416 = And(x=w723, y=w695) -> (x .and. y?=→"bHasMached":bool)
    n417 = Compound Arithmetic op=AND(w475, w476, w477, w478) -> (w474:bool)
    n418 = And(x=w525, y=w474) -> (x .and. y?=w524:bool)
    n419 = And(x=w602, y=w524) -> (x .and. y?=w492:bool)
    n420 = Compound Arithmetic op=AND(w501, w500, w499, w498, w497, w496, w495) -> (w494:bool)
    n421 = Not(x=w494) -> (.not. x?=w493:bool)
    n422 = And(x=w493, y=w492) -> (x .and. y?=w491:bool)
    n423 = And(x=w626, y=w491) -> (x .and. y?=w627:bool)
    n424 = And(x=w735, y=w627) -> (x .and. y?=w734:bool)
    n425 = And(x=w733, y=w734) -> (x .and. y?=w732:bool)
    n426 = And(x=w731, y=w732) -> (x .and. y?=w730:bool)
    n427 = And(x=w729, y=w730) -> (x .and. y?=w728:bool)
    n428 = And(x=w727, y=w728) -> (x .and. y?=w726:bool)
    n429 = And(x=w725, y=w726) -> (x .and. y?=w724:bool)
    n430 = And(x=w737, y=w724) -> (x .and. y?=w736:bool)
    n431 = And(x=w738, y=w736) -> (x .and. y?=→"Write Status":bool)
    n432 = feedback #2(TRUE) -> (w547:bool)
    n433 = And(x=w547, y=w550) -> (x .and. y?=w549:bool)
    n434 = feedback #3(TRUE) -> (w557:bool)
    n435 = And(x=w557, y=w560) -> (x .and. y?=w559:bool)
    n436 = feedback #4(TRUE) -> (w561:bool)
    n437 = And(x=w561, y=w564) -> (x .and. y?=w563:bool)
    n438 = feedback #5(TRUE) -> (w553:bool)
    n439 = And(x=w553, y=w552) -> (x .and. y?=w554:bool)
    n440 = case shown="False" w554 {
      tunnel: [w1239 FALSE] -> w544
      tunnel: w545 -> [w1241 _]
      frame False {
        n441 = Or(x=w1241, y=FALSE) -> (x .or. y?=w1239:bool)
      }
      frame True {
        n442 = call "Charge relay error"() -> ()  [unwired: 10 in, 2 out]
      }
    }
    n443 = feedback-in #5(w544) -> ()
    n444 = case shown="False" w549 {
      tunnel: [w1237 FALSE] -> w548
      tunnel: w544 -> [w1235 _]
      frame False {
        n445 = Or(x=w1235, y=FALSE) -> (x .or. y?=w1237:bool)
      }
      frame True {
        n446 = call "PSU HV error"() -> ()  [unwired: 10 in, 2 out]
      }
    }
    n447 = feedback-in #2(w548) -> ()
    n448 = case shown="False" w563 {
      tunnel: [w1248 FALSE] -> w562
      tunnel: w545 -> [w1247 _]
      frame False {
        n449 = Or(x=w1247, y=FALSE) -> (x .or. y?=w1248:bool)
      }
      frame True {
        n450 = call "Softdump error"() -> ()  [unwired: 10 in, 2 out]
      }
    }
    n451 = feedback-in #4(w562) -> ()
    n452 = case shown="False" w559 {
      tunnel: [w1243 FALSE] -> w558
      tunnel: w544 -> [w1244 _]
      frame False {
        n453 = Or(x=w1244, y=FALSE) -> (x .or. y?=w1243:bool)
      }
      frame True {
        n454 = call "Soft Exception"() -> ()  [unwired: 10 in, 2 out]
      }
    }
    n455 = feedback-in #3(w558) -> ()
    n456 = Compound Arithmetic op=OR(w648, w694, w693) -> (w692:bool)
    n457 = Compound Arithmetic op=OR(w692, w691, w690) -> (w689:bool)
    n458 = Compound Arithmetic op=OR(w689, w688, w687) -> (w686:bool)
    n459 = Compound Arithmetic op=OR(w686, w685, w684) -> (w683:bool)
    n460 = Compound Arithmetic op=OR(w683, w682, w681) -> (w680:bool)
    n461 = Compound Arithmetic op=OR(w680, w679, w678) -> (w677:bool)
    n462 = Compound Arithmetic op=OR(w677, w676, w675) -> (w674:bool)
    n463 = Compound Arithmetic op=OR(w674, w673, w672) -> (w623:bool)
    n464 = Compound Arithmetic op=OR(w623, w625, w624) -> (w591:bool)
    n465 = Compound Arithmetic op=OR(w591, w671, w670) -> (w669:bool)
    n466 = Compound Arithmetic op=OR(w669, w668, w667) -> (w666:bool)
    n467 = Compound Arithmetic op=OR(w666, w665, w664) -> (w663:bool)
    n468 = Compound Arithmetic op=OR(w663, w662, w661) -> (w660:bool)
    n469 = Compound Arithmetic op=OR(w660, w659, w658) -> (w657:bool)
    n470 = Compound Arithmetic op=OR(w657, w656, w655) -> (w654:bool)
    n471 = Compound Arithmetic op=OR(w654, w653, w652) -> (w651:bool)
    n472 = Compound Arithmetic op=OR(w651, w650, w649) -> (w603:bool)
    n473 = Compound Arithmetic op=OR(w603, w601, w600) -> (w593:bool)
    n474 = Compound Arithmetic op=OR(w593, "EXIT HMI", w791) -> (w589:bool)
    "Stop Loops" <- w589
    n475 = property on="Stop Loops" class="Bool (strict)"("Val(Sgnl)"=w589) -> ()  [unwired: 2 in, 2 out]
    n476 = node-c288() -> ()  [unwired: 1 in, 1 out]
  }
  n477 = node-c288(w97) -> (w95:errorcluster)
  n478 = call <userlib>:"Release Writer.vi"("Handle"=w211, "WriteHandle"=w210, "error in (no error)"=w209) -> ("error out"=w205:errorcluster)  [unwired: 11 in, 1 out]
  n479 = call <userlib>:"Release Writer.vi"("Handle"=w307, "WriteHandle"=w306, "error in (no error)"=w305) -> ("error out"=w313:errorcluster)  [unwired: 11 in, 1 out]
  n480 = call <userlib>:"Release Writer.vi"("Handle"=w287, "WriteHandle"=w286, "error in (no error)"=w285) -> ("error out"=w281:errorcluster)  [unwired: 11 in, 1 out]
  n481 = call <userlib>:"Release Writer.vi"("Handle"=w249, "WriteHandle"=w248, "error in (no error)"=w247) -> ("error out"=w243:errorcluster)  [unwired: 11 in, 1 out]
  n482 = call <userlib>:"Release Type.vi"("Handle"=w208, "TypeHandle"=w207, "error in (no error)"=w206) -> ("error out"=w204:errorcluster)  [unwired: 11 in, 1 out]
  n483 = call <userlib>:"Release Type.vi"("Handle"=w302, "TypeHandle"=w303, "error in (no error)"=w304) -> ("error out"=w314:errorcluster)  [unwired: 11 in, 1 out]
  n484 = call <userlib>:"Release Type.vi"("Handle"=w284, "TypeHandle"=w283, "error in (no error)"=w282) -> ("error out"=w280:errorcluster)  [unwired: 11 in, 1 out]
  n485 = call <userlib>:"Release Writer.vi"("Handle"=w268, "WriteHandle"=w267, "error in (no error)"=w266) -> ("error out"=w262:errorcluster)  [unwired: 11 in, 1 out]
  n486 = call <userlib>:"Release Type.vi"("Handle"=w246, "TypeHandle"=w245, "error in (no error)"=w244) -> ("error out"=w242:errorcluster)  [unwired: 11 in, 1 out]
  n487 = call <userlib>:"Release Writer.vi"("Handle"=w230, "WriteHandle"=w229, "error in (no error)"=w228) -> ("error out"=w224:errorcluster)  [unwired: 11 in, 1 out]
  n488 = call <userlib>:"Release Type.vi"("Handle"=w265, "TypeHandle"=w264, "error in (no error)"=w263) -> ("error out"=w261:errorcluster)  [unwired: 11 in, 1 out]
  n489 = call <userlib>:"Release Type.vi"("Handle"=w227, "TypeHandle"=w226, "error in (no error)"=w225) -> ("error out"=w223:errorcluster)  [unwired: 11 in, 1 out]
  n490 = call <userlib>:"Release Writer.vi"("Handle"=w456, "WriteHandle"=w455, "error in (no error)"=w467) -> ("error out"=w135:errorcluster)  [unwired: 11 in, 1 out]
  n491 = call <userlib>:"Release Writer.vi"("Handle"=w325, "WriteHandle"=w324, "error in (no error)"=w323) -> ("error out"=w319:errorcluster)  [unwired: 11 in, 1 out]
  n492 = call <userlib>:"Release Writer.vi"("Handle"=w421, "WriteHandle"=w420, "error in (no error)"=w419) -> ("error out"=w427:errorcluster)  [unwired: 11 in, 1 out]
  n493 = call <userlib>:"Release Writer.vi"("Handle"=w401, "WriteHandle"=w400, "error in (no error)"=w399) -> ("error out"=w395:errorcluster)  [unwired: 11 in, 1 out]
  n494 = call <userlib>:"Release Writer.vi"("Handle"=w363, "WriteHandle"=w362, "error in (no error)"=w361) -> ("error out"=w357:errorcluster)  [unwired: 11 in, 1 out]
  n495 = call <userlib>:"Release Type.vi"("Handle"=w322, "TypeHandle"=w321, "error in (no error)"=w320) -> ("error out"=w318:errorcluster)  [unwired: 11 in, 1 out]
  n496 = call <userlib>:"Release Type.vi"("Handle"=w416, "TypeHandle"=w417, "error in (no error)"=w418) -> ("error out"=w428:errorcluster)  [unwired: 11 in, 1 out]
  n497 = call <userlib>:"Release Type.vi"("Handle"=w398, "TypeHandle"=w397, "error in (no error)"=w396) -> ("error out"=w394:errorcluster)  [unwired: 11 in, 1 out]
  n498 = call <userlib>:"Release Writer.vi"("Handle"=w382, "WriteHandle"=w381, "error in (no error)"=w380) -> ("error out"=w376:errorcluster)  [unwired: 11 in, 1 out]
  n499 = call <userlib>:"Release Type.vi"("Handle"=w360, "TypeHandle"=w359, "error in (no error)"=w358) -> ("error out"=w356:errorcluster)  [unwired: 11 in, 1 out]
  n500 = call <userlib>:"Release Writer.vi"("Handle"=w344, "WriteHandle"=w343, "error in (no error)"=w342) -> ("error out"=w338:errorcluster)  [unwired: 11 in, 1 out]
  n501 = call <userlib>:"Release Type.vi"("Handle"=w379, "TypeHandle"=w378, "error in (no error)"=w377) -> ("error out"=w375:errorcluster)  [unwired: 11 in, 1 out]
  n502 = call <userlib>:"Release Type.vi"("Handle"=w341, "TypeHandle"=w340, "error in (no error)"=w339) -> ("error out"=w337:errorcluster)  [unwired: 11 in, 1 out]
  n503 = call <userlib>:"Release Writer.vi"("Handle"=w439, "WriteHandle"=w438, "error in (no error)"=w437) -> ("error out"=w433:errorcluster)  [unwired: 11 in, 1 out]
  n504 = call <userlib>:"Release Writer.vi"("Handle"=w79, "WriteHandle"=w78, "error in (no error)"=w77) -> ("error out"=w93:errorcluster)  [unwired: 11 in, 1 out]
  n505 = call <userlib>:"Release Writer.vi"("Handle"=w173, "WriteHandle"=w172, "error in (no error)"=w174) -> ("error out"=w180:errorcluster)  [unwired: 11 in, 1 out]
  n506 = call <userlib>:"Release Type.vi"("Handle"=w436, "TypeHandle"=w435, "error in (no error)"=w434) -> ("error out"=w432:errorcluster)  [unwired: 11 in, 1 out]
  n507 = call <userlib>:"Release Type.vi"("Handle"=w75, "TypeHandle"=w74, "error in (no error)"=w76) -> ("error out"=w92:errorcluster)  [unwired: 11 in, 1 out]
  n508 = call <userlib>:"Release Type.vi"("Handle"=w167, "TypeHandle"=w166, "error in (no error)"=w168) -> ("error out"=w179:errorcluster)  [unwired: 11 in, 1 out]
  n509 = call <userlib>:"Release Writer.vi"("Handle"=w105, "WriteHandle"=w104, "error in (no error)"=w103) -> ("error out"=w107:errorcluster)  [unwired: 11 in, 1 out]
  n510 = call <userlib>:"Release Type.vi"("Handle"=w100, "TypeHandle"=w101, "error in (no error)"=w102) -> ("error out"=w106:errorcluster)  [unwired: 11 in, 1 out]
  n511 = call <userlib>:"Release Writer.vi"("Handle"=w61, "WriteHandle"=w60, "error in (no error)"=w59) -> ("Handle"=w46:u32, "error out"=w71:errorcluster)  [unwired: 11 in]
  n512 = call <userlib>:"Release Type.vi"("Handle"=w57, "TypeHandle"=w56, "error in (no error)"=w58) -> ("error out"=w70:errorcluster)  [unwired: 11 in, 1 out]
  n513 = call <userlib>:"Release Type.vi"("Handle"=w454, "TypeHandle"=w453, "error in (no error)"=w466) -> ("error out"=w136:errorcluster)  [unwired: 11 in, 1 out]
  n514 = Merge Errors(w313, w314) -> (w124:errorcluster)
  n515 = Merge Errors(w205, w204) -> (w119:errorcluster)
  n516 = Merge Errors(w281, w280) -> (w123:errorcluster)
  n517 = Merge Errors(w243, w242) -> (w121:errorcluster)
  n518 = Merge Errors(w262, w261) -> (w122:errorcluster)
  n519 = Merge Errors(w224, w223) -> (w120:errorcluster)
  n520 = Merge Errors(w427, w428) -> (w130:errorcluster)
  n521 = Merge Errors(w319, w318) -> (w125:errorcluster)
  n522 = Merge Errors(w395, w394) -> (w129:errorcluster)
  n523 = Merge Errors(w357, w356) -> (w127:errorcluster)
  n524 = Merge Errors(w376, w375) -> (w128:errorcluster)
  n525 = Merge Errors(w338, w337) -> (w126:errorcluster)
  n526 = Merge Errors(w433, w432) -> (w131:errorcluster)
  n527 = Merge Errors(w93, w92) -> (w91:errorcluster)
  n528 = Merge Errors(w180, w179) -> (w118:errorcluster)
  n529 = Merge Errors(w107, w106) -> (w99:errorcluster)
  n530 = Merge Errors(w71, w70) -> (w55:errorcluster)
  n531 = Merge Errors(w135, w136) -> (w134:errorcluster)
  n532 = Merge Errors(w26, w25, w24, w23, w14) -> (w21:errorcluster)
  n533 = Merge Errors(w130, w129, w128, w127, w126, w125, w91) -> (w197:errorcluster)
  n534 = Merge Errors(w124, w123, w122, w121, w120, w119, w118, w99, w55, w8, w7, w6, w2) -> (w196:errorcluster)
  n535 = Merge Errors(w146, w147, w148, w149, w150, w52, w51, w47, w48, w49, w50) -> (w137:errorcluster)
  n536 = Merge Errors(w94, w145, w144, w143, w142, w141, w140, w139, w37, w36, w35, w22, w21) -> (w138:errorcluster)
  n537 = Merge Errors(w137, w138) -> (w1:errorcluster)
  n538 = Merge Errors(w95, w134, w131, w197, w196, w1) -> (w132:errorcluster)
  n539 = call <userlib>:"Release.vi"("Handle"=w46, "error in (no error)"=w132) -> ("error out"=→"error out":errorcluster)  [unwired: 13 in]
